vi "Periodic Tasks.vi"(8 "error in":errorcluster) -> ()   [LabVIEW 2020]
doc: "This VI runs in parallel to other tasks. It can contain as many user-defined periodic loops as you need. These can carry out PID or other sorts of timed response."
uses:
  Global Variables/Climber_States.ctl
  <vilib>/Rock Robotics/WPI/Solenoid/WPI_SolenoidValue.ctl
  <vilib>/Rock Robotics/WPI/ThirdParty/REV Robotics/REVLib/Typedef/Spark MAX Control Type.ctl
  <vilib>/Rock Robotics/WPI/ThirdParty/Phoenix-LabVIEW/Motor Controller/Controls/CTRE_Phoenix_MotorControl_ControlMode.ctl
  <vilib>/Rock Robotics/WPI/DriverStation/WPI_DriverStationRobotMode2.ctl
  <vilib>/Rock Robotics/WPI/ThirdParty/Phoenix-LabVIEW/Motor Controller/Controls/CTRE_Phoenix_MotorControl_FeedbackDevice.ctl
  Global Variables/Ball_Routine_States.ctl
  Global Variables/Verification_Delay.ctl
  Global Variables/Shooter_States.ctl
  LabVIEW_is_Under_Control.lib/Util/Toggle/Change Detect.vi
  LabVIEW_is_Under_Control.lib/Util/Toggle/Change Detect Boolean.vi
  <vilib>/Rock Robotics/WPI/Utilities/WPI_GetSetVariantRefNum.vi
  Global Variables/Axes_N_Buttons.vi
  Global Variables/ActuatorsSensors.vi
  Global Variables/StateMachineOperation.vi
  <vilib>/Rock Robotics/Network Tables/NT Write Number.vi
  <vilib>/Rock Robotics/WPI/Solenoid/WPI_SolenoidSetEnum.vi
  Robot Global Data.vi
  <vilib>/Rock Robotics/WPI/ThirdParty/Phoenix-LabVIEW/Motor Controller/Get/CTRE_Phoenix_MotorController_GetSelectedSensorData.vi
  <vilib>/Rock Robotics/Network Tables/NT Write Boolean.vi
  <vilib>/Rock Robotics/Network Tables/NT Write String.vi
panel:
  in  "Robot Control":T1(tab)=enum."Shooter"
  out "Right Current":dbl
  out "Left Current":dbl
  out "Left Current":T2(graph)
  in  "Sensitivity":dbl=1.1
  out "Right Current":T2(graph)
  in  "Reset L":bool
  in  "Reset R":bool
  out "Sensor Position R":dbl=13.714309692382812
  out "Sensor Position L":dbl=5.142850875854492
  out "Shooting?":bool
  out "Applied Output":dbl
  out "ShooterRPM":dbl=352.7285869172389
  out "Voltage":dbl=12.2890625
  out "Output":cluster{"Voltage":dbl}(graph)
  out "Setpoint Shooter":dbl=850.0
  out "PID":cluster{"Setpoint":dbl, "Sensor Position":dbl}(graph)={"Setpoint"=0.0, "Sensor Position"=352.7285869172389}
  in  "PID Constants":T3={"P Gain"=1.5e-05, "I Gain"=0.0, "D Gain"=0.0, "F Gain"=0.00022, "I Zone"=100000.0, "Min Output"=-1.0, "Max Output"=1.0}
  out "RPM Ready?":bool
  in  "SpShooter":dbl=850.0
  in  "Gains":T4={"proportional gain (Kc)"=0.0005, "integral time (Ti, min)"=0.005, "derivative time (Td, min)"=0.0} {"derivative time (Td, min)" format="%.6f"; "integral time (Ti, min)" format="%.6f"; "proportional gain (Kc)" format="%.6f"}
  in  "Range":cluster{"output high":dbl, "output low":dbl}={"output high"=1.0, "output low"=0.0} {"output low" format="%.2f"; "output high" format="%.2f"}
  in  "SpShooter Low Goal":dbl=1000.0
  in  "Hood Low Goal SP":dbl=1000.0
  out "ShooterHoodRPM;":dbl=-0.0
  out "Waveform Chart Hood":cluster{"Shooter Setpoint":dbl, dbl}(graph)={"Shooter Setpoint"=3000.0, -0.0}
  out "Output Chart Hood":cluster{"Percent Output":dbl}(graph)
  in  "I Zone Hood":dbl=1000.0
  in  "kF Hood":dbl=0.005
  in  "D Hood":dbl
  in  "I Hood":dbl
  in  "P Hood":dbl=0.0045
  in  "Neutral to Full Seconds Hood":dbl
  in  "Hood Setpoint Shooter":dbl=3000.0
  out "Setpoint Shooter Hood":dbl=3000.0
  in  "Reset Climber":bool
  out "Climbing State":T5
  out "Climbing?":bool
  out "Sensor Position":dbl
  out "1 Ball only":bool
  out "Discard Left":bool
  out "Discard Right":bool
  out "Overwrite Solenoid":bool
  out "Has 2 Balls":bool
  out "Left Infrared Conveyor":bool
  out "Right Infrared Conveyor":bool
  out "Has Ball Left":bool
  out "Has Ball Right":bool
  out "Opposite Ball Right":bool
  out "Opposite Ball Left":bool
  out "Opposite Color":string="Red"
  out "Ball Color":string="Blue"
  out "RightColor":u32(colorbox)=4488510
  out "LeftColor":u32(colorbox)=4488765
  out "Left Switch Conveyor":bool
  out "Right Switch Conveyor":bool
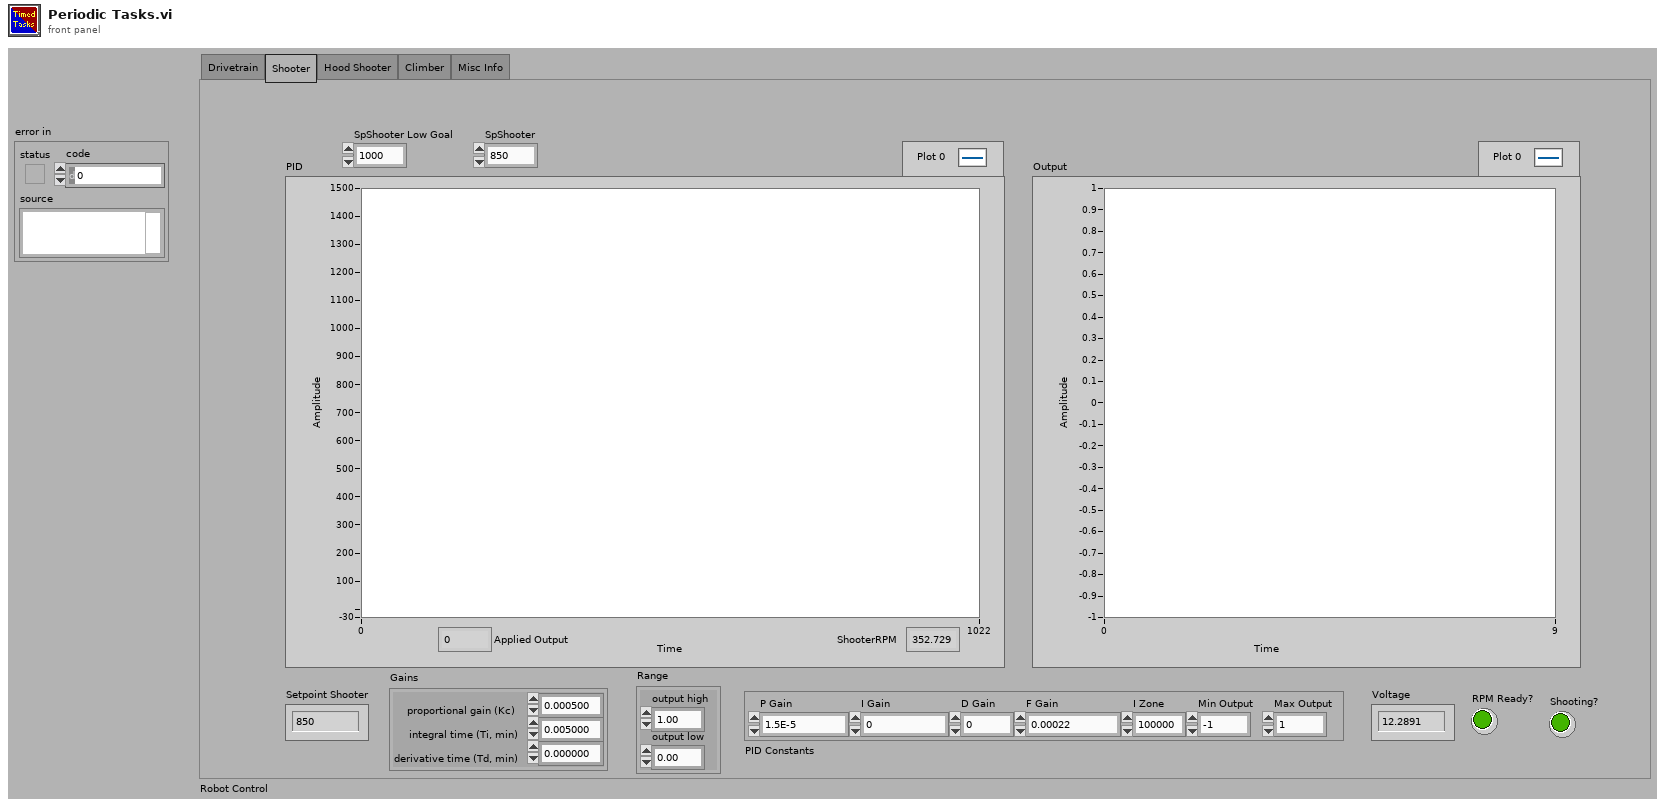
[diagram p1: front panel]
types:
  T1 = enum32{"Drivetrain", "Shooter", "Hood Shooter", "Climber", "Misc Info"}
  T2 = cluster{"current (A)":dbl, "current (A)":dbl, "current (A)":dbl}
  T3 = cluster{"P Gain":dbl, "I Gain":dbl, "D Gain":dbl, "F Gain":dbl, "I Zone":dbl, "Min Output":dbl, "Max Output":dbl}
  T4 = cluster{"proportional gain (Kc)":dbl, "integral time (Ti, min)":dbl, "derivative time (Td, min)":dbl}
  T5 = typedef "Climber_States.ctl" = enum16{"Start Lock", "Release Climber", "Reset Encoder", "Pull Climber", "Lock Pull", "Final Pull", "Lock", "Unspool Release"}
  T6 = typedef "WPI_MotorControlDeviceRef.ctl" = cluster{"DeviceStatus":errorcluster, "Type":T7, "PWM":cluster{"PWM Channel":T8, "DeadBand":T9}, "CAN":cluster{"Device Number":u8, "SetOutput VI Ref":variant, "GetOutput VI Ref":variant, "Enable VI Ref":variant, "Disable VI Ref":variant, "Data":variant}, "Invert":bool, "DIO PWM":cluster{"PWM \"Enable\" Channel":T8, "DIOChannel":T10, "PWM Rate":dbl}}
  T7 = typedef "WPI_MotorControlType.ctl" = enum16{"PWM", "CAN", "DIO PWM"}
  T8 = typedef "FPGA_DIOPWMChannel.ctl" = enum8{"PWM 0", "PWM 1", "PWM 2", "PWM 3", "PWM 4", "PWM 5", "PWM 6", "PWM 7", "PWM 8", "PWM 9", "PWM MXP 0", "PWM MXP 1", "PWM MXP 2", "PWM MXP 3", "PWM MXP 4", "PWM MXP 5", "PWM MXP 6", "PWM MXP 7", "PWM MXP 8", "PWM MXP 9", "Invalid"}
  T9 = typedef "WPI_PWMDeadband.ctl" = cluster{"Name":string, "maxPositivePwm":i32, "minPositivePwm":i32, "centerPwm":i32, "maxNegativePwm":i32, "minNegativePwm":i32, "angularRange":u16}
  T10 = typedef "FPGA_DIOChannel.ctl" = enum8{"DIO 0", "DIO 1", "DIO 2", "DIO 3", "DIO 4", "DIO 5", "DIO 6", "DIO 7", "DIO 8", "DIO 9", "DIO MXP 0", "DIO MXP 1", "DIO MXP 2", "DIO MXP 3", "DIO MXP 4", "DIO MXP 5", "DIO MXP 6", "DIO MXP 7", "DIO MXP 8", "DIO MXP 9", "DIO MXP 10", "DIO MXP 11", "DIO MXP 12", "DIO MXP 13", "DIO MXP 14", "DIO MXP 15", "SPI Port CS1", "SPI Port CS2", "SPI Port CS3", "SPI Port MISO", "SPI Port MOSI", "Invalid"}
  T11 = typedef "WPI_SwitchDevRef.ctl" = cluster{"DevStatus":errorcluster, "DIO Channel":T10, "CntIndex":T12, "Normally Closed":bool}
  T12 = typedef "FPGA_CounterCtrSystemIndex.ctl" = enum8{"Ctr 0", "Ctr 1", "Ctr 2", "Ctr 3", "Ctr 4", "Ctr 5", "Ctr 6", "Ctr 7", "Invalid"}
  T13 = typedef "WPI_DigitalOutputDevRef.ctl" = cluster{"DIO Channel":T10, "DevStatus":errorcluster}
  T14 = typedef "WPI_SolenoidDevRef.ctl" = cluster{"DevStatus":errorcluster, "Pneumatics Control Module":u8, "Forward Solenoid Channel":T15, "Reverse Solenoid Channel":T15}
  T15 = typedef "WPI_SolenoidChannel.ctl" = enum8{"Solenoid 0", "Solenoid 1", "Solenoid 2", "Solenoid 3", "Solenoid 4", "Solenoid 5", "Solenoid 6", "Solenoid 7", "Solenoid 8", "Solenoid 9", "Solenoid 10", "Solenoid 11", "Solenoid 12", "Solenoid 13", "Solenoid 14", "Solenoid 15", "Invalid"}
  T16 = typedef "WPI_CompressorDevRef.ctl" = cluster{"DevStatus":errorcluster, "Pneumatics Control Module":u8}
  T17 = typedef "WPI_SolenoidValue.ctl" = enum16{"Off", "On", "Forward", "Reverse"}
  T18 = typedef "Spark MAX Control Type.ctl" = enum16{"Percent VBus", "Voltage", "Velocity", "Position", "Smart Motion", "Current", "Smart Velocity"}
  T19 = typedef "CTRE_Phoenix_MotorControl_ControlMode.ctl" = u16
  T20 = typedef "WPI_DriverStationRobotMode2.ctl" = enum16{"Autonomous Disabled", "Autonomous Enabled", "Teleop Disabled", "Teleop Enabled", "Disconnected", "Finish", "Test Disabled", "Test Enabled", "Emergency Stopped"}
  T21 = typedef "Color Sensor V3 DevRef.ctl" = cluster{"I2CDevRef":T22}
  T22 = typedef "WPI_I2CDevRef.ctl" = cluster{"DevStatus":errorcluster, "Device Address":u8, "Handle":i32, "I2C Bus":T23}
  T23 = typedef "i2c_bus.ctl" = enum16{"I2C On-Board", "I2C MXP", "Invalid"}
  T24 = typedef "Verification_Delay.ctl" = enum16{"Verifying", "Delayed"}
  T25 = typedef "Ball_Routine_States.ctl" = enum16{"Default", "Dual Intake Collect", "Front Intake Collect", "Rear Intake Collect", "Prepare Shooter", "Shoot", "Climbing", "Opposite Ball Detected", "Low Goal Mode", "Low Goal Shoot"}
  T26 = typedef "WPI_EncoderDevRef.ctl" = cluster{"DevStatus":errorcluster, "EncoderIndex":T27, "CounterIndex":T12, "DistancePerCount":dbl, "Decoding Type":T28}
  T27 = typedef "FPGA_EncoderIdx.ctl" = enum8{"Enc 0", "Enc 1", "Enc 2", "Enc 3", "Enc 4", "Enc 5", "Enc 6", "Enc 7", "Invalid"}
  T28 = typedef "WPI_EncoderType.ctl" = enum16{"1x", "2x", "4x"}
  T29 = typedef "CTRE_Phoenix_MotorControl_FeedbackDevice.ctl" = i8
  T30 = typedef "Shooter_States.ctl" = enum16{"Disabled", "Cruise Velocity", "Shooting Velocity"}
  T31 = cluster{"P Gain":bool, "I Gain":bool, "D Gain":bool, "F Gain":bool, "I Zone":bool, "Min Output":bool, "Max Output":bool}
  T32 = cluster{"Setpoint Shooter":dbl, "Sensor Velocity":dbl}
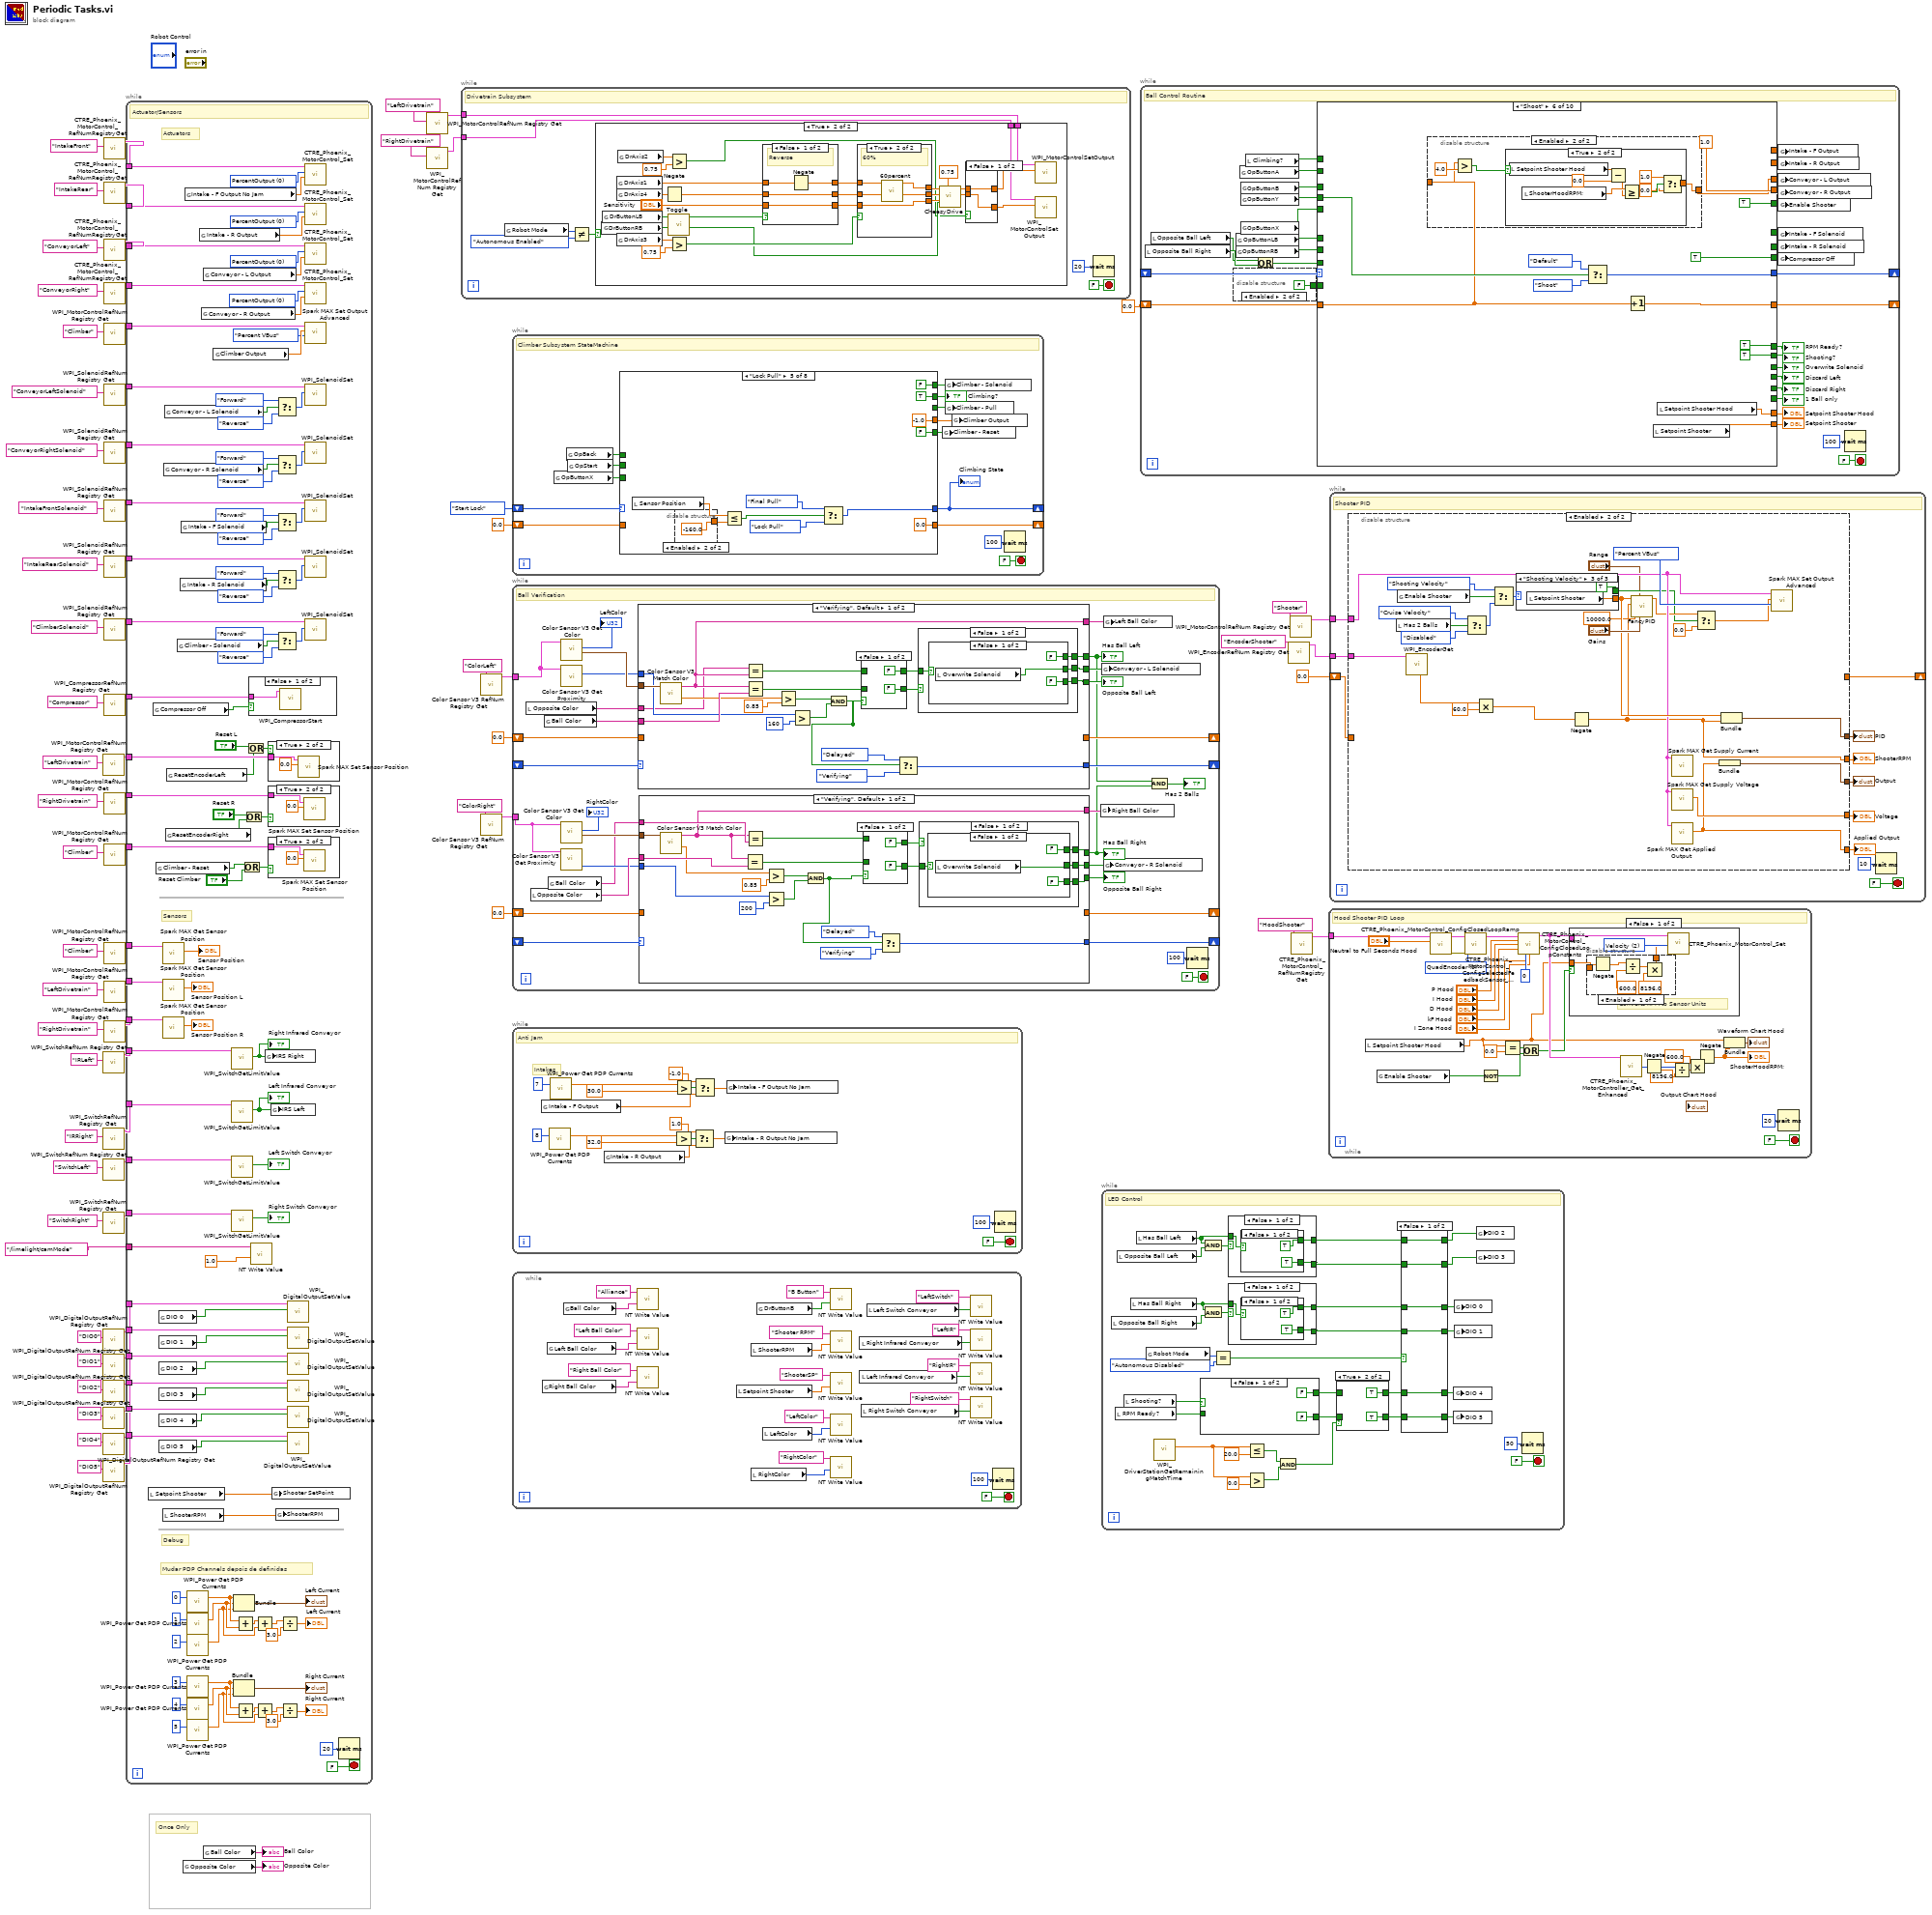
[diagram p0: block diagram]
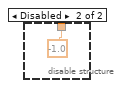
[diagram p2: hidden frame]
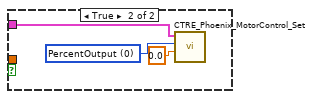
[diagram p3: hidden frame]
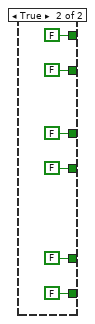
[diagram p4: hidden frame]
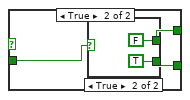
[diagram p6: hidden frame]
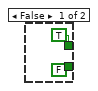
[diagram p7: hidden frame]
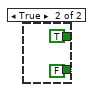
[diagram p8: hidden frame]
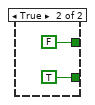
[diagram p9: hidden frame]
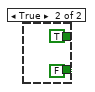
[diagram p10: hidden frame]
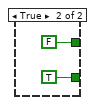
[diagram p11: hidden frame]
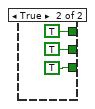
[diagram p13: hidden frame]
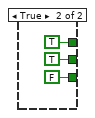
[diagram p14: hidden frame]
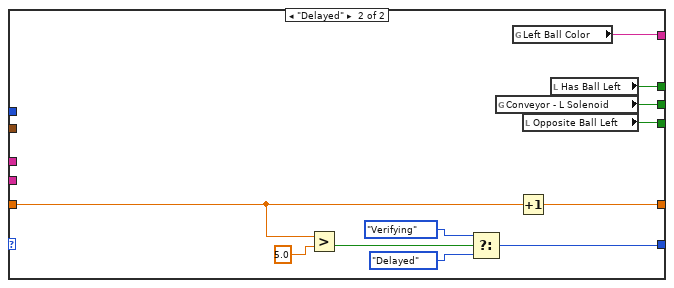
[diagram p15: hidden frame]
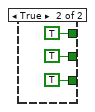
[diagram p17: hidden frame]
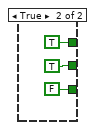
[diagram p18: hidden frame]
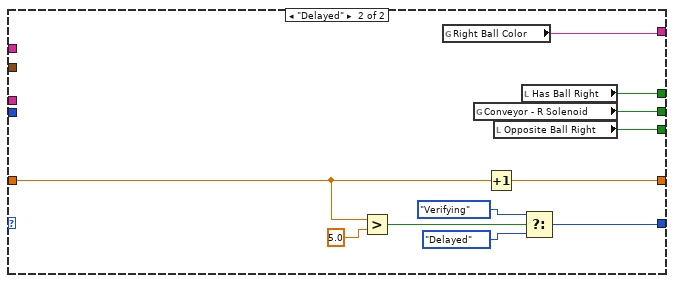
[diagram p19: hidden frame]
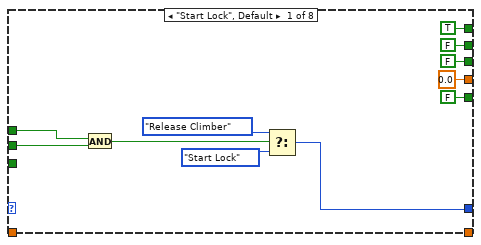
[diagram p20: hidden frame]
diagram:
  # "Once Only"
  n1 = call <vilib>:"WPI_MotorControlRefNum Registry Get.vi"("refnum name"="LeftDrivetrain") -> ("MotorControlDevRef"=w53:T6)  [unwired: 9 in, 1 out]
  n2 = call <vilib>:"WPI_SwitchRefNum Registry Get.vi"("refnum name"="IRLeft") -> ("SwitchDevRef"=w57:T11)  [unwired: 9 in, 1 out]
  n3 = call <vilib>:"WPI_SwitchRefNum Registry Get.vi"("refnum name"="IRRight") -> ("SwitchDevRef"=w56:T11)  [unwired: 9 in, 1 out]
  n4 = call <vilib>:"WPI_SwitchRefNum Registry Get.vi"("refnum name"="SwitchLeft") -> ("SwitchDevRef"=w38:T11)  [unwired: 9 in, 1 out]
  n5 = call <vilib>:"WPI_SwitchRefNum Registry Get.vi"("refnum name"="SwitchRight") -> ("SwitchDevRef"=w37:T11)  [unwired: 9 in, 1 out]
  n6 = call <vilib>:"WPI_DigitalOutputRefNum Registry Get.vi"("refnum name"="DIO0") -> ("DigitalOutputDevRef"=w21:T13)  [unwired: 9 in, 1 out]
  n7 = call <vilib>:"WPI_DigitalOutputRefNum Registry Get.vi"("refnum name"="DIO1") -> ("DigitalOutputDevRef"=w14:T13)  [unwired: 9 in, 1 out]
  n8 = call <vilib>:"WPI_DigitalOutputRefNum Registry Get.vi"("refnum name"="DIO2") -> ("DigitalOutputDevRef"=w13:T13)  [unwired: 9 in, 1 out]
  n9 = call <vilib>:"WPI_DigitalOutputRefNum Registry Get.vi"("refnum name"="DIO3") -> ("DigitalOutputDevRef"=w12:T13)  [unwired: 9 in, 1 out]
  n10 = call <vilib>:"WPI_DigitalOutputRefNum Registry Get.vi"("refnum name"="DIO4") -> ("DigitalOutputDevRef"=w11:T13)  [unwired: 9 in, 1 out]
  n11 = call <vilib>:"WPI_DigitalOutputRefNum Registry Get.vi"("refnum name"="DIO5") -> ("DigitalOutputDevRef"=w10:T13)  [unwired: 9 in, 1 out]
  n12 = call <vilib>:"CTRE_Phoenix_MotorControl_RefNumRegistryGet.vi"("refnum name"="IntakeFront") -> ("PhoenixMotorControlDevRef"=w77:T6)  [unwired: 9 in, 1 out]
  n13 = call <vilib>:"CTRE_Phoenix_MotorControl_RefNumRegistryGet.vi"("refnum name"="IntakeRear") -> ("PhoenixMotorControlDevRef"=w75:T6)  [unwired: 9 in, 1 out]
  n14 = call <vilib>:"CTRE_Phoenix_MotorControl_RefNumRegistryGet.vi"("refnum name"="ConveyorLeft") -> ("PhoenixMotorControlDevRef"=w74:T6)  [unwired: 9 in, 1 out]
  n15 = call <vilib>:"CTRE_Phoenix_MotorControl_RefNumRegistryGet.vi"("refnum name"="ConveyorRight") -> ("PhoenixMotorControlDevRef"=w71:T6)  [unwired: 9 in, 1 out]
  n16 = call <vilib>:"WPI_MotorControlRefNum Registry Get.vi"("refnum name"="Climber") -> ("MotorControlDevRef"=w70:T6)  [unwired: 9 in, 1 out]
  n17 = call <vilib>:"WPI_SolenoidRefNum Registry Get.vi"("refnum name"="ConveyorLeftSolenoid") -> ("SolenoidDevRef"=w69:T14)  [unwired: 9 in, 1 out]
  n18 = call <vilib>:"WPI_SolenoidRefNum Registry Get.vi"("refnum name"="ConveyorRightSolenoid") -> ("SolenoidDevRef"=w68:T14)  [unwired: 9 in, 1 out]
  n19 = call <vilib>:"WPI_SolenoidRefNum Registry Get.vi"("refnum name"="IntakeFrontSolenoid") -> ("SolenoidDevRef"=w67:T14)  [unwired: 9 in, 1 out]
  n20 = call <vilib>:"WPI_SolenoidRefNum Registry Get.vi"("refnum name"="IntakeRearSolenoid") -> ("SolenoidDevRef"=w60:T14)  [unwired: 9 in, 1 out]
  n21 = call <vilib>:"WPI_SolenoidRefNum Registry Get.vi"("refnum name"="ClimberSolenoid") -> ("SolenoidDevRef"=w66:T14)  [unwired: 9 in, 1 out]
  n22 = call <vilib>:"WPI_CompressorRefNum Registry Get.vi"("refnum name"="Compressor") -> ("CompressorDevRef"=w55:T16)  [unwired: 9 in, 1 out]
  n23 = call <vilib>:"WPI_MotorControlRefNum Registry Get.vi"("refnum name"="RightDrivetrain") -> ("MotorControlDevRef"=w54:T6)  [unwired: 9 in, 1 out]
  n24 = call <vilib>:"WPI_MotorControlRefNum Registry Get.vi"("refnum name"="Climber") -> ("MotorControlDevRef"=w48:T6)  [unwired: 9 in, 1 out]
  n25 = call <vilib>:"WPI_MotorControlRefNum Registry Get.vi"("refnum name"="Climber") -> ("MotorControlDevRef"=w46:T6)  [unwired: 9 in, 1 out]
  n26 = call <vilib>:"WPI_MotorControlRefNum Registry Get.vi"("refnum name"="LeftDrivetrain") -> ("MotorControlDevRef"=w40:T6)  [unwired: 9 in, 1 out]
  n27 = call <vilib>:"WPI_MotorControlRefNum Registry Get.vi"("refnum name"="RightDrivetrain") -> ("MotorControlDevRef"=w39:T6)  [unwired: 9 in, 1 out]
  n28 = while {
    tunnel: w77 -> [w183]
    tunnel: w75 -> [w180]
    tunnel: w74 -> [w179]
    tunnel: w71 -> [w178]
    tunnel: w70 -> [w177]
    tunnel: w69 -> [w176]
    tunnel: w68 -> [w175]
    tunnel: w67 -> [w174]
    tunnel: w66 -> [w173]
    tunnel: w60 -> [w168]
    tunnel: w57 -> [w137]
    tunnel: w56 -> [w136]
    tunnel: w55 -> [w134]
    tunnel: w54 -> [w132]
    tunnel: w53 -> [w131]
    tunnel: w48 -> [w130]
    tunnel: w46 -> [w129]
    tunnel: w40 -> [w122]
    tunnel: w39 -> [w121]
    tunnel: w38 -> [w112]
    tunnel: w37 -> [w111]
    tunnel: "/limelight/camMode" ("Name") -> [w99]
    tunnel: w21 -> [w90]
    tunnel: w14 -> [w89]
    tunnel: w13 -> [w88]
    tunnel: w12 -> [w87]
    tunnel: w11 -> [w86]
    tunnel: w10 -> [w85]
    stop <- FALSE stop-if-true
    w93 = T19 0 items=["PercentOutput"=0, "Position"=1, "Velocity"=2, "Current"=3, "Follower"=5, "MotionProfile"=6, "MotionMagic"=7, "MotionProfileArc"=10, "Disabled"=15] ("Control Mode")
    w94 = T19 0 items=["PercentOutput"=0, "Position"=1, "Velocity"=2, "Current"=3, "Follower"=5, "MotionProfile"=6, "MotionMagic"=7, "MotionProfileArc"=10, "Disabled"=15] ("Control Mode")
    w102 = T19 0 items=["PercentOutput"=0, "Position"=1, "Velocity"=2, "Current"=3, "Follower"=5, "MotionProfile"=6, "MotionMagic"=7, "MotionProfileArc"=10, "Disabled"=15] ("Control Mode")
    w181 = T19 0 items=["PercentOutput"=0, "Position"=1, "Velocity"=2, "Current"=3, "Follower"=5, "MotionProfile"=6, "MotionMagic"=7, "MotionProfileArc"=10, "Disabled"=15] ("Control Mode")
    # "Debug"
    # "Mudar PDP Channels depois de definidas"
    # "Sensors"
    # "Actuators"
    # "Actuator/Sensors"
    n29 = local read "Setpoint Shooter"() -> (w78:dbl)
    n30 = global read "ActuatorsSensors.vi" "Compressor Off"() -> (w133:bool)
    n31 = global read "StateMachineOperation.vi" "Climber - Reset"() -> (w124:bool)
    n32 = global read "ActuatorsSensors.vi" "DIO 0"() -> (w84:bool)
    n33 = global read "ActuatorsSensors.vi" "DIO 1"() -> (w83:bool)
    n34 = global read "ActuatorsSensors.vi" "DIO 2"() -> (w82:bool)
    n35 = global read "ActuatorsSensors.vi" "DIO 3"() -> (w81:bool)
    n36 = global read "ActuatorsSensors.vi" "DIO 4"() -> (w80:bool)
    n37 = global read "ActuatorsSensors.vi" "DIO 5"() -> (w79:bool)
    n38 = call <vilib>:"Spark MAX Get Sensor Position.vi"("MotorControlDevRef in"=w129) -> ("Sensor Position"=→"Sensor Position":dbl)  [unwired: 7 in, 3 out]
    n39 = call <vilib>:"Spark MAX Get Sensor Position.vi"("MotorControlDevRef in"=w122) -> ("Sensor Position"=→"Sensor Position L":dbl)  [unwired: 7 in, 3 out]
    n40 = call <vilib>:"Spark MAX Get Sensor Position.vi"("MotorControlDevRef in"=w121) -> ("Sensor Position"=→"Sensor Position R":dbl)  [unwired: 7 in, 3 out]
    n41 = local read "ShooterRPM"() -> (w135:dbl)
    n42 = global read "ActuatorsSensors.vi" "Conveyor - R Solenoid"() -> (w139:bool)
    n43 = global read "ActuatorsSensors.vi" "Conveyor - L Solenoid"() -> (w138:bool)
    n44 = global read "ActuatorsSensors.vi" "ResetEncoderRight"() -> (w118:bool)
    n45 = global read "ActuatorsSensors.vi" "ResetEncoderLeft"() -> (w114:bool)
    n46 = global read "ActuatorsSensors.vi" "Climber - Solenoid"() -> (w107:bool)
    n47 = global read "ActuatorsSensors.vi" "Intake - R Solenoid"() -> (w104:bool)
    n48 = global read "ActuatorsSensors.vi" "Intake - F Solenoid"() -> (w169:bool)
    n49 = global read "ActuatorsSensors.vi" "Intake - F Output No Jam"() -> (w182:dbl)
    n50 = call <vilib>:"WPI_Power Get PDP Currents.vi"("PDP Channel"=0) -> ("current (A)"=w163:dbl)  [unwired: 12 in, 2 out]
    n51 = call <vilib>:"WPI_Power Get PDP Currents.vi"("PDP Channel"=1) -> ("current (A)"=w162:dbl)  [unwired: 12 in, 2 out]
    n52 = call <vilib>:"WPI_Power Get PDP Currents.vi"("PDP Channel"=2) -> ("current (A)"=w160:dbl)  [unwired: 12 in, 2 out]
    n53 = call <vilib>:"WPI_Power Get PDP Currents.vi"("PDP Channel"=3) -> ("current (A)"=w155:dbl)  [unwired: 12 in, 2 out]
    n54 = call <vilib>:"WPI_Power Get PDP Currents.vi"("PDP Channel"=4) -> ("current (A)"=w154:dbl)  [unwired: 12 in, 2 out]
    n55 = call <vilib>:"WPI_Power Get PDP Currents.vi"("PDP Channel"=5) -> ("current (A)"=w152:dbl)  [unwired: 12 in, 2 out]
    n56 = global read "ActuatorsSensors.vi" "Intake - R Output"() -> (w101:dbl)
    n57 = global read "ActuatorsSensors.vi" "Conveyor - R Output"() -> (w91:dbl)
    n58 = global read "ActuatorsSensors.vi" "Conveyor - L Output"() -> (w92:dbl)
    n59 = global read "ActuatorsSensors.vi" "Climber Output"() -> (w127:dbl)
    n60 = call <vilib>:"WPI_SwitchGetLimitValue.vi"("SwitchDevRef"=w137) -> ("Switch Pressed"=w98:bool)  [unwired: 8 in, 2 out]
    "Right Infrared Conveyor" <- w98
    n61 = call <vilib>:"WPI_SwitchGetLimitValue.vi"("SwitchDevRef"=w136) -> ("Switch Pressed"=w97:bool)  [unwired: 8 in, 2 out]
    "Left Infrared Conveyor" <- w97
    n62 = call <vilib>:"WPI_SwitchGetLimitValue.vi"("SwitchDevRef"=w112) -> ("Switch Pressed"=→"Left Switch Conveyor":bool)  [unwired: 8 in, 2 out]
    n63 = call <vilib>:"WPI_SwitchGetLimitValue.vi"("SwitchDevRef"=w111) -> ("Switch Pressed"=→"Right Switch Conveyor":bool)  [unwired: 8 in, 2 out]
    n64 = Bundle("current (A)"=w163, "current (A)"=w162, "current (A)"=w160) -> (→"Left Current":T2)  [unwired: 1 in]
    n65 = Bundle("current (A)"=w155, "current (A)"=w154, "current (A)"=w152) -> (→"Right Current":T2)  [unwired: 1 in]
    n66 = Add(x=w163, y=w162) -> (x+y=w161:dbl)
    n67 = Add(x=w155, y=w154) -> (x+y=w153:dbl)
    n68 = Or(x=w124, y="Reset Climber") -> (x .or. y?=w126:bool)
    n69 = Or(x="Reset R", y=w118) -> (x .or. y?=w117:bool)
    n70 = Or(x="Reset L", y=w114) -> (x .or. y?=w115:bool)
    n71 = case shown="False" w133 {
      tunnel: w134 -> [w192 w193]
      frame False {
        n72 = call <vilib>:"WPI_CompressorStart.vi"("CompressorDevRef"=w192) -> ()  [unwired: 9 in, 2 out]
      }
      frame True {
        n73 = call <vilib>:"WPI_CompressorStop.vi"("CompressorDevRef"=w193) -> ()  [unwired: 9 in, 2 out]
      }
    }
    n74 = call-poly <vilib>:"NT Write Value.vi"("Numeric"=1.0, "Name"=w99) -> ()  [unwired: 9 in, 1 out]
    n75 = Add(x=w161, y=w160) -> (x+y=w159:dbl)
    n76 = Add(x=w153, y=w152) -> (x+y=w151:dbl)
    n77 = global write "ActuatorsSensors.vi" "IRS Right"(w98) -> ()
    n78 = case shown="True" w115 {
      tunnel: w131 -> [_ w188]
      frame False {
      }
      frame True {
        n79 = call <vilib>:"Spark MAX Set Sensor Position.vi"("Position"=0.0, "MotorControlDeviceRef"=w188) -> ()  [unwired: 8 in, 2 out]
      }
    }
    n80 = case shown="True" w117 {
      tunnel: w132 -> [_ w190]
      frame False {
      }
      frame True {
        n81 = call <vilib>:"Spark MAX Set Sensor Position.vi"("Position"=0.0, "MotorControlDeviceRef"=w190) -> ()  [unwired: 8 in, 2 out]
      }
    }
    n82 = case shown="True" w126 {
      tunnel: w130 -> [_ w186]
      frame False {
      }
      frame True {
        n83 = call <vilib>:"Spark MAX Set Sensor Position.vi"("Position"=0.0, "MotorControlDeviceRef"=w186) -> ()  [unwired: 8 in, 2 out]
      }
    }
    n84 = global write "ActuatorsSensors.vi" "IRS Left"(w97) -> ()
    n85 = global write "ActuatorsSensors.vi" "Shooter SetPoint"(w78) -> ()
    n86 = global write "ActuatorsSensors.vi" "ShooterRPM"(w135) -> ()
    n87 = Select(t=WPI_SolenoidValue."Forward" ("Value"), s=w138, f=WPI_SolenoidValue."Reverse" ("Value")) -> (s? t:f=w141:T17)
    n88 = Select(t=WPI_SolenoidValue."Forward" ("Value"), s=w139, f=WPI_SolenoidValue."Reverse" ("Value")) -> (s? t:f=w140:T17)
    n89 = Select(t=WPI_SolenoidValue."Forward" ("Value"), s=w169, f=WPI_SolenoidValue."Reverse" ("Value")) -> (s? t:f=w170:T17)
    n90 = Select(t=WPI_SolenoidValue."Forward" ("Value"), s=w104, f=WPI_SolenoidValue."Reverse" ("Value")) -> (s? t:f=w103:T17)
    n91 = Select(t=WPI_SolenoidValue."Forward" ("Value"), s=w107, f=WPI_SolenoidValue."Reverse" ("Value")) -> (s? t:f=w108:T17)
    n92 = Divide(x=w159, y=3.0) -> (x/y=→"Left Current":dbl)
    n93 = Divide(x=w151, y=3.0) -> (x/y=→"Right Current":dbl)
    n94 = call <vilib>:"WPI_DigitalOutputSetValue.vi"("Value"=w84, "DigitalOutputDevRef"=w90) -> ()  [unwired: 8 in, 2 out]
    n95 = call <vilib>:"WPI_DigitalOutputSetValue.vi"("Value"=w83, "DigitalOutputDevRef"=w89) -> ()  [unwired: 8 in, 2 out]
    n96 = call <vilib>:"WPI_DigitalOutputSetValue.vi"("Value"=w82, "DigitalOutputDevRef"=w88) -> ()  [unwired: 8 in, 2 out]
    n97 = call <vilib>:"WPI_DigitalOutputSetValue.vi"("Value"=w81, "DigitalOutputDevRef"=w87) -> ()  [unwired: 8 in, 2 out]
    n98 = call <vilib>:"WPI_DigitalOutputSetValue.vi"("Value"=w80, "DigitalOutputDevRef"=w86) -> ()  [unwired: 8 in, 2 out]
    n99 = call <vilib>:"WPI_DigitalOutputSetValue.vi"("Value"=w79, "DigitalOutputDevRef"=w85) -> ()  [unwired: 8 in, 2 out]
    n100 = call <vilib>:"CTRE_Phoenix_MotorControl_Set.vi"("Output"=w182, "Control Mode"=w181, "PhoenixMotorControlDevRef"=w183) -> ()  [unwired: 7 in, 2 out]
    n101 = call <vilib>:"CTRE_Phoenix_MotorControl_Set.vi"("Output"=w101, "Control Mode"=w102, "PhoenixMotorControlDevRef"=w180) -> ()  [unwired: 7 in, 2 out]
    n102 = call <vilib>:"CTRE_Phoenix_MotorControl_Set.vi"("Output"=w92, "Control Mode"=w93, "PhoenixMotorControlDevRef"=w179) -> ()  [unwired: 7 in, 2 out]
    n103 = call <vilib>:"CTRE_Phoenix_MotorControl_Set.vi"("Output"=w91, "Control Mode"=w94, "PhoenixMotorControlDevRef"=w178) -> ()  [unwired: 7 in, 2 out]
    n104 = call <vilib>:"Spark MAX Set Output Advanced.vi"("Control Mode"=Spark_MAX_Control_Type."Percent VBus", "Setpoint"=w127, "MotorControlDevRef"=w177) -> ()  [unwired: 7 in, 2 out]
    n105 = call-poly <vilib>:"WPI_SolenoidSet.vi"("Value"=w141, "SolenoidDevRef"=w176) -> ()  [unwired: 8 in, 2 out]
    n106 = call-poly <vilib>:"WPI_SolenoidSet.vi"("Value"=w140, "SolenoidDevRef"=w175) -> ()  [unwired: 8 in, 2 out]
    n107 = call-poly <vilib>:"WPI_SolenoidSet.vi"("Value"=w170, "SolenoidDevRef"=w174) -> ()  [unwired: 8 in, 2 out]
    n108 = call-poly <vilib>:"WPI_SolenoidSet.vi"("Value"=w103, "SolenoidDevRef"=w168) -> ()  [unwired: 8 in, 2 out]
    n109 = call-poly <vilib>:"WPI_SolenoidSet.vi"("Value"=w108, "SolenoidDevRef"=w173) -> ()  [unwired: 8 in, 2 out]
    n110 = Wait (ms)(milliseconds to wait=u32 20) -> ()  [unwired: 1 out]
  }
  n111 = global read "StateMachineOperation.vi" "Opposite Color"() -> (→"Opposite Color":string)
  n112 = global read "StateMachineOperation.vi" "Ball Color"() -> (→"Ball Color":string)
  n113 = call <vilib>:"WPI_MotorControlRefNum Registry Get.vi"("refnum name"="LeftDrivetrain") -> ("MotorControlDevRef"=w6:T6)  [unwired: 9 in, 1 out]
  n114 = call <vilib>:"WPI_MotorControlRefNum Registry Get.vi"("refnum name"="RightDrivetrain") -> ("MotorControlDevRef"=w5:T6)  [unwired: 9 in, 1 out]
  n115 = while {
    tunnel: w6 -> [w195]
    tunnel: w5 -> [w194]
    stop <- FALSE stop-if-true
    # "Drivetrain Subsystem"
    n116 = global read "Robot Global Data.vi" "Robot Mode"() -> (w198:T20)
    n117 = Not Equal?(x=w198, y=WPI_DriverStationRobotMode2."Autonomous Enabled" ("Robot Mode")) -> (x != y?=w196:bool)
    n118 = case shown="True" w196 {
      tunnel: w195 -> [_ w211]
      tunnel: w194 -> [_ w202]
      frame False {
      }
      frame True {
        n119 = global read "Axes_N_Buttons.vi" "DrButtonRB"() -> (w212:bool)
        n120 = global read "Axes_N_Buttons.vi" "DrButtonLB"() -> (w224:bool)
        n121 = global read "Axes_N_Buttons.vi" "DrAxis1"() -> (w207:dbl)
        n122 = global read "Axes_N_Buttons.vi" "DrAxis4"() -> (w225:dbl)
        n123 = global read "Axes_N_Buttons.vi" "DrAxis3"() -> (w215:dbl)
        n124 = global read "Axes_N_Buttons.vi" "DrAxis2"() -> (w210:dbl)
        n125 = Negate(x=w225) -> (-x=w208:dbl)
        n126 = call "Toggle.vi"("In"=w224) -> ("Toggled"=w223:bool)  [unwired: 10 in]
        n127 = Greater?(x=w215, y=0.75) -> (0:w213:bool)
        n128 = Greater?(x=w210, y=0.75) -> (0:w206:bool)
        n129 = case shown="False" w223 {
          tunnel: w207 -> [w240 w242]
          tunnel: w208 -> [w239 w243]
          tunnel: "Sensitivity" -> [w241 w244]
          tunnel: [w241 w244] -> w221
          tunnel: [w238 w242] -> w219
          tunnel: [w239 w243] -> w220
          frame False {
            # "Reverse"
            n130 = Negate(x=w240) -> (-x=w238:dbl)
          }
          frame True {
            # "Reverse"
          }
        }
        n131 = case shown="True" w213 {
          tunnel: w221 -> [w231 w237]
          tunnel: w220 -> [w232 w236]
          tunnel: w219 -> [w233 w235]
          tunnel: [w231 w237] -> w218
          tunnel: [w232 w236] -> w217
          tunnel: [w233 w234] -> w216
          frame False {
            # "60%"
          }
          frame True {
            # "60%"
            n132 = call "60percent.vi"("In"=w235) -> ("Out"=w234:dbl)  [unwired: 10 in]
          }
        }
        n133 = call "CheesyDrive.vi"("Quickturn"=w212, "WheelNonLinearity"=0.75, "Sensitivty"=w218, "Wheel"=w217, "Throttle"=w216) -> ("Right PWM"=w204:dbl, "Left PWM"=w205:dbl)  [unwired: 5 in]
        n134 = case shown="False" w206 {
          tunnel: w205 -> [w228 _]
          tunnel: w204 -> [w227 _]
          tunnel: [w228 0.06 ("Left PWM")] -> w203
          tunnel: [w227 0.06 ("Right PWM")] -> w201
          frame False {
          }
          frame True {
          }
        }
        n135 = call <vilib>:"WPI_MotorControlSetOutput.vi"("Output"=w203, "MotorControlDevRef"=w211) -> ()  [unwired: 7 in, 3 out]
        n136 = call <vilib>:"WPI_MotorControlSetOutput.vi"("Output"=w201, "MotorControlDevRef"=w202) -> ()  [unwired: 7 in, 3 out]
      }
    }
    n137 = Wait (ms)(milliseconds to wait=u32 20) -> ()  [unwired: 1 out]
  }
  n138 = call <vilib>:"Color Sensor V3 RefNum Registry Get.vi"("refnum name"="ColorLeft") -> ("ColorSensorDevRef"=w30:T21)  [unwired: 9 in, 1 out]
  n139 = call <vilib>:"Color Sensor V3 RefNum Registry Get.vi"("refnum name"="ColorRight") -> ("ColorSensorDevRef"=w29:T21)  [unwired: 9 in, 1 out]
  n140 = while {
    shift-right: [w253] -> _
    shift-left: Climber_States."Start Lock" ("Enum") -> [w255]
    shift-right: [w245] -> _
    shift-left: 0.0 ("y") -> [w246]
    stop <- FALSE stop-if-true
    # "Climber Subsystem StateMachine"
    n141 = global read "Axes_N_Buttons.vi" "OpButtonX"() -> (w251:bool)
    n142 = global read "Axes_N_Buttons.vi" "OpBack"() -> (w256:bool)
    n143 = global read "Axes_N_Buttons.vi" "OpStart"() -> (w249:bool)
    n144 = case shown="\"Lock Pull\"" w255 {
      tunnel: w256 -> [w269 _ _ _ _ _ w327 _]
      tunnel: [TRUE ("ClimberSolenoid") FALSE ("ClimberSolenoid") _ FALSE ("ClimberSolenoid") FALSE ("ClimberSolenoid") TRUE ("ClimberSolenoid") TRUE ("ClimberSolenoid") FALSE ("ClimberSolenoid")] -> w252
      tunnel: [FALSE ("Climbing?") TRUE ("Climbing?") TRUE ("Climbing?") TRUE ("Climbing?") TRUE ("Climbing?") TRUE ("Climbing?") FALSE ("Climbing?") TRUE ("Climbing?")] -> w254
      tunnel: [w265 w273 w281 w292 w307 w320 w325 w337] -> w253
      tunnel: w251 -> [_ w272 _ _ _ _ _ w338]
      tunnel: [FALSE FALSE _ TRUE _ _ _ _] -> w250
      tunnel: w249 -> [w261 _ _ _ _ _ w326 _]
      tunnel: [0.0 ("y") _ _ -1.0 ("OpAxis1") -1.0 ("OpAxis1") -1.0 ("OpAxis1") 0.0 ("OpAxis1") w344] -> w248
      tunnel: [FALSE ("Climber - Pull") FALSE ("Climber - Pull") TRUE ("Climber - Pull") FALSE ("Climber - Pull") FALSE ("Climber - Pull") FALSE ("Climber - Pull") FALSE ("Climber - Pull") FALSE ("Climber - Pull")] -> w247
      tunnel: [_ _ w285 _ 0.0 w322 _ _] -> w245
      tunnel: w246 -> [_ _ w284 _ _ w321 _ _]
      frame "Start Lock", Default {
        n145 = And(x=w269, y=w261) -> (x .and. y?=w268:bool)
        n146 = Select(t=Climber_States."Release Climber" ("Enum"), s=w268, f=Climber_States."Start Lock" ("Enum")) -> (s? t:f=w265:T5)
      }
      frame "Release Climber" {
        n147 = Select(t=Climber_States."Reset Encoder" ("Enum"), s=w272, f=Climber_States."Release Climber" ("Enum")) -> (s? t:f=w273:T5)
      }
      frame "Reset Encoder" {
        n148 = Greater?(x=w284, y=1.0) -> (0:w282:bool)
        n149 = Increment(x=w284) -> (x+1=w285:dbl)
        n150 = Select(t=Climber_States."Pull Climber" ("Enum"), s=w282, f=Climber_States."Reset Encoder" ("Enum")) -> (s? t:f=w281:T5)
      }
      frame "Pull Climber" {
        n151 = local read "Sensor Position"() -> (w291:dbl)
        n152 = disable-structure shown="Enabled" {
          disable-tunnel: [-99.0 ("y") -115.0 ("y")] -> w288
          frame Disabled {
          }
          frame Enabled {
          }
        }
        n153 = Less Or Equal?(x=w291, y=w288) -> (x <= y?=w290:bool)
        n154 = Select(t=Climber_States."Lock Pull" ("Enum"), s=w290, f=Climber_States."Pull Climber" ("Enum")) -> (s? t:f=w292:T5)
      }
      frame "Lock Pull" {
        n155 = local read "Sensor Position"() -> (w309:dbl)
        n156 = disable-structure shown="Enabled" {
          disable-tunnel: [-122.5 ("y") -160.0 ("y")] -> w308
          frame Disabled {
          }
          frame Enabled {
          }
        }
        n157 = Less Or Equal?(x=w309, y=w308) -> (x <= y?=w304:bool)
        n158 = Select(t=Climber_States."Final Pull" ("Enum"), s=w304, f=Climber_States."Lock Pull" ("Enum")) -> (s? t:f=w307:T5)
      }
      frame "Final Pull" {
        n159 = Greater?(x=w321, y=1.0) -> (0:w319:bool)
        n160 = Select(t=Climber_States."Lock" ("Enum"), s=w319, f=Climber_States."Final Pull" ("Enum")) -> (s? t:f=w320:T5)
        n161 = Increment(x=w321) -> (x+1=w322:dbl)
      }
      frame "Lock" {
        n162 = And(x=w327, y=w326) -> (x .and. y?=w330:bool)
        n163 = Select(t=Climber_States."Unspool Release" ("Enum"), s=w330, f=Climber_States."Lock" ("Enum")) -> (s? t:f=w325:T5)
      }
      frame "Unspool Release" {
        n164 = local read "Sensor Position"() -> (w347:dbl)
        n165 = local read "Sensor Position"() -> (w349:dbl)
        n166 = Greater Or Equal?(x=w349, y=-1.0) -> (x >= y?=w336:bool)
        n167 = Greater Or Equal?(x=w347, y=-10.0) -> (x >= y?=w335:bool)
        n168 = Select(t=0.2, s=w335, f=1.0) -> (s? t:f=w343:dbl)
        n169 = Select(t=Climber_States."Reset Encoder" ("Enum"), s=w338, f=Climber_States."Unspool Release" ("Enum")) -> (s? t:f=w337:T5)
        n170 = Select(t=0.0, s=w336, f=w343) -> (s? t:f=w344:dbl)
      }
    }
    "Climbing?" <- w254
    "Climbing State" <- w253
    n171 = global write "StateMachineOperation.vi" "Climber - Reset"(w247) -> ()
    n172 = global write "ActuatorsSensors.vi" "Climber - Solenoid"(w252) -> ()
    n173 = global write "StateMachineOperation.vi" "Climber - Pull"(w250) -> ()
    n174 = global write "ActuatorsSensors.vi" "Climber Output"(w248) -> ()
    n175 = Wait (ms)(milliseconds to wait=u32 100) -> ()  [unwired: 1 out]
  }
  n176 = while {
    tunnel: w30 -> [w373]
    tunnel: w29 -> [w372]
    shift-right: [w374] -> _
    shift-left: _ -> [w364]
    shift-right: [w362] -> _
    shift-left: 0.0 ("y") -> [w363]
    shift-right: [w357] -> _
    shift-left: _ -> [w358]
    shift-right: [w355] -> _
    shift-left: 0.0 ("y") -> [w356]
    stop <- FALSE stop-if-true
    # "Ball Verification"
    n177 = local read "Opposite Color"() -> (w361:string)
    n178 = local read "Opposite Color"() -> (w377:string)
    n179 = global read "StateMachineOperation.vi" "Ball Color"() -> (w378:string)
    n180 = global read "StateMachineOperation.vi" "Ball Color"() -> (w360:string)
    n181 = call <vilib>:"Color Sensor V3 Get Color.vi"("ColorSensorDevRef"=w372) -> ("Normalized Color"=w375:cluster{"R":dbl, "G":dbl, "B":dbl}, "Color"=→"RightColor":u32)  [unwired: 7 in, 2 out]
    n182 = call <vilib>:"Color Sensor V3 Get Proximity.vi"("ColorSensorDevRef"=w372) -> ("Proximity"=w371:u16)  [unwired: 8 in, 2 out]
    n183 = call <vilib>:"Color Sensor V3 Get Color.vi"("ColorSensorDevRef"=w373) -> ("Normalized Color"=w376:cluster{"R":dbl, "G":dbl, "B":dbl}, "Color"=→"LeftColor":u32)  [unwired: 7 in, 2 out]
    n184 = call <vilib>:"Color Sensor V3 Get Proximity.vi"("ColorSensorDevRef"=w373) -> ("Proximity"=w370:u16)  [unwired: 8 in, 2 out]
    n185 = case shown="\"Verifying\", Default" w358 {
      tunnel: w378 -> [w403 _]
      tunnel: w376 -> [w402 _]
      tunnel: w370 -> [w401 _]
      tunnel: [w400 w423] -> w368
      tunnel: [w399 w424] -> w367
      tunnel: [w398 w422] -> w352
      tunnel: [w392 w425] -> w365
      tunnel: w361 -> [w388 _]
      tunnel: [w383 w426] -> w357
      tunnel: [_ w431] -> w355
      tunnel: w356 -> [_ w427]
      frame "Verifying", Default {
        n186 = call <vilib>:"Color Sensor V3 Match Color.vi"("Measured Color"=w402) -> ("Confidence"=w397:dbl, "Matched Color Name"=w392:string)  [unwired: 8 in, 1 out]
        n187 = Equal?(x=w388, y=w392) -> (x = y?=w393:bool)
        n188 = Equal?(x=w392, y=w403) -> (x = y?=w395:bool)
        n189 = Greater?(x=w397, y=0.85) -> (0:w389:bool)
        n190 = Greater?(x=w401, y=u16 160) -> (0:w387:bool)
        n191 = And(x=w389, y=w387) -> (x .and. y?=w384:bool)
        n192 = case shown="False" w384 {
          tunnel: [FALSE w407] -> w394
          tunnel: w393 -> [_ w407]
          tunnel: w395 -> [_ w406]
          tunnel: [FALSE w406] -> w396
          frame False {
          }
          frame True {
          }
        }
        n193 = Select(t=Verification_Delay."Delayed" ("Verification Delay State"), s=w384, f=Verification_Delay."Verifying" ("Verification Delay State")) -> (s? t:f=w383:T24)
        n194 = case shown="False" w396 {
          tunnel: w394 -> [w411 _]
          tunnel: [w409 FALSE ("Opposite Ball?")] -> w400
          tunnel: [w410 TRUE ("Conveyor - L Solenoid")] -> w399
          tunnel: [w408 TRUE ("Has Ball Left")] -> w398
          frame False {
            n195 = case shown="False" w411 {
              tunnel: [w412 TRUE ("Conveyor - L Solenoid")] -> w410
              tunnel: [FALSE ("Opposite Ball?") TRUE ("Opposite Ball?")] -> w409
              tunnel: [FALSE ("Has Ball Left") TRUE ("Has Ball Left")] -> w408
              frame False {
                n196 = local read "Overwrite Solenoid"() -> (w412:bool)
              }
              frame True {
              }
            }
          }
          frame True {
          }
        }
      }
      frame "Delayed" {
        n197 = Greater?(x=w427, y=5.0) -> (0:w429:bool)
        n198 = Select(t=Verification_Delay."Verifying" ("Verification Delay State"), s=w429, f=Verification_Delay."Delayed" ("Verification Delay State")) -> (s? t:f=w426:T24)
        n199 = global read "ActuatorsSensors.vi" "Conveyor - L Solenoid"() -> (w424:bool)
        n200 = global read "StateMachineOperation.vi" "Left Ball Color"() -> (w425:string)
        n201 = Increment(x=w427) -> (x+1=w431:dbl)
        n202 = local read "Opposite Ball Left"() -> (w423:bool)
        n203 = local read "Has Ball Left"() -> (w422:bool)
      }
    }
    "Opposite Ball Left" <- w368
    "Has Ball Left" <- w352
    n204 = case shown="\"Verifying\", Default" w364 {
      tunnel: w377 -> [w452 _]
      tunnel: w375 -> [w451 _]
      tunnel: [w450 w474] -> w374
      tunnel: w371 -> [w449 _]
      tunnel: [w448 w472] -> w369
      tunnel: [w447 w470] -> w366
      tunnel: [w446 w471] -> w353
      tunnel: [_ w480] -> w362
      tunnel: w363 -> [_ w479]
      tunnel: w360 -> [w434 _]
      tunnel: [w432 w473] -> w359
      frame "Verifying", Default {
        n205 = call <vilib>:"Color Sensor V3 Match Color.vi"("Measured Color"=w451) -> ("Confidence"=w441:dbl, "Matched Color Name"=w432:string)  [unwired: 8 in, 1 out]
        n206 = Equal?(x=w432, y=w452) -> (x = y?=w444:bool)
        n207 = Equal?(x=w432, y=w434) -> (x = y?=w442:bool)
        n208 = Greater?(x=w441, y=0.85) -> (0:w437:bool)
        n209 = Greater?(x=w449, y=u16 200) -> (0:w435:bool)
        n210 = And(x=w437, y=w435) -> (x .and. y?=w433:bool)
        n211 = case shown="False" w433 {
          tunnel: [FALSE w456] -> w443
          tunnel: w442 -> [_ w456]
          tunnel: [FALSE w455] -> w445
          tunnel: w444 -> [_ w455]
          frame False {
          }
          frame True {
          }
        }
        n212 = Select(t=Verification_Delay."Delayed" ("Verification Delay State"), s=w433, f=Verification_Delay."Verifying" ("Verification Delay State")) -> (s? t:f=w450:T24)
        n213 = case shown="False" w443 {
          tunnel: w445 -> [w460 _]
          tunnel: [w459 TRUE ("Conveyor - L Solenoid")] -> w448
          tunnel: [w458 FALSE ("Opposite Ball?")] -> w447
          tunnel: [w457 TRUE ("Has Ball Right")] -> w446
          frame False {
            n214 = case shown="False" w460 {
              tunnel: [w461 TRUE ("Conveyor - L Solenoid")] -> w459
              tunnel: [FALSE ("Opposite Ball?") TRUE ("Opposite Ball?")] -> w458
              tunnel: [FALSE ("Has Ball Right") TRUE ("Has Ball Right")] -> w457
              frame False {
                n215 = local read "Overwrite Solenoid"() -> (w461:bool)
              }
              frame True {
              }
            }
          }
          frame True {
          }
        }
      }
      frame "Delayed" {
        n216 = Greater?(x=w479, y=5.0) -> (0:w477:bool)
        n217 = global read "StateMachineOperation.vi" "Right Ball Color"() -> (w473:string)
        n218 = global read "ActuatorsSensors.vi" "Conveyor - R Solenoid"() -> (w472:bool)
        n219 = Increment(x=w479) -> (x+1=w480:dbl)
        n220 = local read "Opposite Ball Right"() -> (w470:bool)
        n221 = local read "Has Ball Right"() -> (w471:bool)
        n222 = Select(t=Verification_Delay."Verifying" ("Verification Delay State"), s=w477, f=Verification_Delay."Delayed" ("Verification Delay State")) -> (s? t:f=w474:T24)
      }
    }
    "Opposite Ball Right" <- w366
    "Has Ball Right" <- w353
    n223 = global write "StateMachineOperation.vi" "Right Ball Color"(w359) -> ()
    n224 = global write "ActuatorsSensors.vi" "Conveyor - L Solenoid"(w367) -> ()
    n225 = global write "ActuatorsSensors.vi" "Conveyor - R Solenoid"(w369) -> ()
    n226 = global write "StateMachineOperation.vi" "Left Ball Color"(w365) -> ()
    n227 = And(x=w352, y=w353) -> (x .and. y?=→"Has 2 Balls":bool)
    n228 = Wait (ms)(milliseconds to wait=u32 100) -> ()  [unwired: 1 out]
  }
  n229 = while {
    stop <- FALSE stop-if-true
    # "Intakes"
    # "Anti Jam"
    n230 = global read "ActuatorsSensors.vi" "Intake - F Output"() -> (w491:dbl)
    n231 = call <vilib>:"WPI_Power Get PDP Currents.vi"("PDP Channel"=8) -> ("current (A)"=w486:dbl)  [unwired: 12 in, 2 out]
    n232 = call <vilib>:"WPI_Power Get PDP Currents.vi"("PDP Channel"=7) -> ("current (A)"=w495:dbl)  [unwired: 12 in, 2 out]
    n233 = global read "ActuatorsSensors.vi" "Intake - R Output"() -> (w482:dbl)
    n234 = Greater?(x=w486, y=32.0) -> (0:w484:bool)
    n235 = Greater?(x=w495, y=30.0) -> (0:w494:bool)
    n236 = Select(t=1.0 ("f"), s=w484, f=w482) -> (s? t:f=w481:dbl)
    n237 = Select(t=-1.0 ("f"), s=w494, f=w491) -> (s? t:f=w490:dbl)
    n238 = global write "ActuatorsSensors.vi" "Intake - R Output No Jam"(w481) -> ()
    n239 = global write "ActuatorsSensors.vi" "Intake - F Output No Jam"(w490) -> ()
    n240 = Wait (ms)(milliseconds to wait=u32 100) -> ()  [unwired: 1 out]
  }
  n241 = while {
    stop <- FALSE stop-if-true
    n242 = global read "StateMachineOperation.vi" "Right Ball Color"() -> (w515:string)
    n243 = global read "StateMachineOperation.vi" "Left Ball Color"() -> (w517:string)
    n244 = global read "StateMachineOperation.vi" "Ball Color"() -> (w519:string)
    n245 = call-poly <vilib>:"NT Write Value.vi"("String"=w519, "Name"="Alliance") -> ()  [unwired: 9 in, 1 out]
    n246 = call-poly <vilib>:"NT Write Value.vi"("String"=w517, "Name"="Left Ball Color") -> ()  [unwired: 9 in, 1 out]
    n247 = call-poly <vilib>:"NT Write Value.vi"("String"=w515, "Name"="Right Ball Color") -> ()  [unwired: 9 in, 1 out]
    n248 = local read "Setpoint Shooter"() -> (w509:dbl)
    n249 = local read "ShooterRPM"() -> (w513:dbl)
    n250 = local read "RightColor"() -> (w506:u32)
    n251 = global read "Axes_N_Buttons.vi" "DrButtonB"() -> (w521:bool)
    n252 = local read "LeftColor"() -> (w508:u32)
    n253 = call-poly <vilib>:"NT Write Value.vi"("Boolean"=w521, "Name"="B Button") -> ()  [unwired: 9 in, 1 out]
    n254 = call-poly <vilib>:"NT Write Value.vi"("Numeric"=w513, "Name"="Shooter RPM") -> ()  [unwired: 9 in, 1 out]
    n255 = call-poly <vilib>:"NT Write Value.vi"("Numeric"=w509, "Name"="ShooterSP") -> ()  [unwired: 9 in, 1 out]
    n256 = call-poly <vilib>:"NT Write Value.vi"("Numeric"=w508, "Name"="LeftColor") -> ()  [unwired: 9 in, 1 out]
    n257 = call-poly <vilib>:"NT Write Value.vi"("Numeric"=w506, "Name"="RightColor") -> ()  [unwired: 9 in, 1 out]
    n258 = local read "Right Infrared Conveyor"() -> (w503:bool)
    n259 = local read "Left Infrared Conveyor"() -> (w502:bool)
    n260 = local read "Right Switch Conveyor"() -> (w501:bool)
    n261 = local read "Left Switch Conveyor"() -> (w504:bool)
    n262 = call-poly <vilib>:"NT Write Value.vi"("Boolean"=w504, "Name"="LeftSwitch") -> ()  [unwired: 9 in, 1 out]
    n263 = call-poly <vilib>:"NT Write Value.vi"("Boolean"=w503, "Name"="LeftIR") -> ()  [unwired: 9 in, 1 out]
    n264 = call-poly <vilib>:"NT Write Value.vi"("Boolean"=w502, "Name"="RightIR") -> ()  [unwired: 9 in, 1 out]
    n265 = call-poly <vilib>:"NT Write Value.vi"("Boolean"=w501, "Name"="RightSwitch") -> ()  [unwired: 9 in, 1 out]
    n266 = Wait (ms)(milliseconds to wait=u32 100) -> ()  [unwired: 1 out]
  }
  n267 = while {
    stop <- FALSE stop-if-true
    # "LED Control"
    n268 = local read "Opposite Ball Right"() -> (w549:bool)
    n269 = local read "RPM Ready?"() -> (w546:bool)
    n270 = local read "Opposite Ball Left"() -> (w552:bool)
    n271 = local read "Shooting?"() -> (w547:bool)
    n272 = local read "Has Ball Right"() -> (w548:bool)
    n273 = local read "Has Ball Left"() -> (w551:bool)
    n274 = global read "Robot Global Data.vi" "Robot Mode"() -> (w525:T20)
    n275 = call <vilib>:"WPI_DriverStationGetRemainingMatchTime.vi"() -> ("Match Time(s)"=w532:sgl)  [unwired: 10 in, 1 out]
    n276 = case shown="False" w547 {
      tunnel: [FALSE ("DIO 4") w576] -> w544
      tunnel: [FALSE ("DIO 5") w575] -> w545
      tunnel: w546 -> [_ w574]
      frame False {
      }
      frame True {
        n277 = case shown="True" w574 {
          tunnel: [TRUE ("DIO 4") FALSE ("DIO 4")] -> w576
          tunnel: [FALSE ("DIO 5") TRUE ("DIO 5")] -> w575
          frame False {
          }
          frame True {
          }
        }
      }
    }
    n278 = And(x=w551, y=w552) -> (x .and. y?=w553:bool)
    n279 = And(x=w548, y=w549) -> (x .and. y?=w550:bool)
    n280 = Equal?(x=w525, y=WPI_DriverStationRobotMode2."Autonomous Disabled" ("Robot Mode")) -> (x = y?=w523:bool)
    n281 = case shown="False" w553 {
      tunnel: [w590 TRUE ("DIO 1")] -> w542
      tunnel: [w591 FALSE ("DIO 0")] -> w543
      tunnel: w551 -> [w592 _]
      frame False {
        n282 = case shown="False" w592 {
          tunnel: [TRUE ("DIO 0") TRUE ("DIO 0")] -> w591
          tunnel: [TRUE ("DIO 1") FALSE ("DIO 1")] -> w590
          frame False {
          }
          frame True {
          }
        }
      }
      frame True {
      }
    }
    n283 = case shown="False" w550 {
      tunnel: [w581 TRUE ("DIO 1")] -> w539
      tunnel: [w582 FALSE ("DIO 0")] -> w541
      tunnel: w548 -> [w583 _]
      frame False {
        n284 = case shown="False" w583 {
          tunnel: [TRUE ("DIO 0") TRUE ("DIO 0")] -> w582
          tunnel: [TRUE ("DIO 1") FALSE ("DIO 1")] -> w581
          frame False {
          }
          frame True {
          }
        }
      }
      frame True {
      }
    }
    n285 = Less Or Equal?(x=w532, y=sgl 20.0) -> (x <= y?=w530:bool)
    n286 = Greater?(x=w532, y=sgl 0.0) -> (0:w529:bool)
    n287 = And(x=w530, y=w529) -> (x .and. y?=w528:bool)
    n288 = case shown="True" w528 {
      tunnel: w545 -> [w569 _]
      tunnel: [w569 TRUE ("DIO 5")] -> w535
      tunnel: w544 -> [w568 _]
      tunnel: [w568 TRUE ("DIO 4")] -> w537
      frame False {
      }
      frame True {
      }
    }
    n289 = case shown="False" w523 {
      tunnel: w543 -> [w560 _]
      tunnel: w542 -> [w561 _]
      tunnel: [w561 FALSE ("DIO 1")] -> w526
      tunnel: [w560 FALSE ("DIO 0")] -> w527
      tunnel: [w559 FALSE ("DIO 0")] -> w540
      tunnel: w541 -> [w559 _]
      tunnel: [w558 FALSE ("DIO 1")] -> w538
      tunnel: w539 -> [w558 _]
      tunnel: [w557 FALSE ("DIO 4")] -> w536
      tunnel: w537 -> [w557 _]
      tunnel: w535 -> [w556 _]
      tunnel: [w556 FALSE ("DIO 5")] -> w534
      frame False {
      }
      frame True {
      }
    }
    n290 = global write "ActuatorsSensors.vi" "DIO 4"(w536) -> ()
    n291 = global write "ActuatorsSensors.vi" "DIO 5"(w534) -> ()
    n292 = global write "ActuatorsSensors.vi" "DIO 0"(w540) -> ()
    n293 = global write "ActuatorsSensors.vi" "DIO 1"(w538) -> ()
    n294 = global write "ActuatorsSensors.vi" "DIO 2"(w527) -> ()
    n295 = global write "ActuatorsSensors.vi" "DIO 3"(w526) -> ()
    n296 = Wait (ms)(milliseconds to wait=u32 50) -> ()  [unwired: 1 out]
  }
  n297 = while {
    shift-right: [w626] -> _
    shift-left: _ -> [w625]
    shift-right: [w610] -> _
    shift-left: 0.0 ("y") -> [w611]
    stop <- FALSE stop-if-true
    # "Ball Control Routine"
    n298 = local read "Opposite Ball Right"() -> (w601:bool)
    n299 = local read "Opposite Ball Left"() -> (w600:bool)
    n300 = disable-structure shown="Enabled" {
      disable-tunnel: [w633 FALSE ("Toggled")] -> w604
      frame Disabled {
        n301 = global read "Axes_N_Buttons.vi" "OpLeft"() -> (w634:bool)
        n302 = call "Toggle.vi"("Initial Value"=FALSE, "In"=w634) -> ("Toggled"=w633:bool)  [unwired: 9 in]
      }
      frame Enabled {
      }
    }
    n303 = global read "Axes_N_Buttons.vi" "OpButtonRB"() -> (w627:bool)
    n304 = global read "Axes_N_Buttons.vi" "OpButtonLB"() -> (w628:bool)
    n305 = global read "Axes_N_Buttons.vi" "OpButtonA"() -> (w631:bool)
    n306 = global read "Axes_N_Buttons.vi" "OpButtonB"() -> (w630:bool)
    n307 = global read "Axes_N_Buttons.vi" "OpButtonY"() -> (w629:bool)
    n308 = global read "Axes_N_Buttons.vi" "OpButtonX"() -> (w616:bool)
    n309 = local read "Climbing?"() -> (w621:bool)
    n310 = Or(x=w600, y=w601) -> (x .or. y?=w599:bool)
    n311 = case shown="\"Shoot\"" w625 {
      tunnel: [w667 _ _ _ w762 w772 _ w824 _ 1.0 ("f")] -> w618
      tunnel: [w667 -1.0 ("Intake Front Output") -1.0 ("Intake Front Output") _ _ _ _ _ _ _] -> w620
      tunnel: w631 -> [w666 _ w699 w716 _ _ _ _ w835 _]
      tunnel: w630 -> [w662 w677 _ w713 _ _ _ _ w834 _]
      tunnel: w629 -> [_ w673 w689 w706 w770 w783 _ _ _ w852]
      tunnel: w628 -> [w659 _ _ _ _ _ _ _ _ _]
      tunnel: w627 -> [_ _ _ _ w761 _ _ _ w831 _]
      tunnel: [w669 w680 w698 w717 w768 w784 w807 w826 w829 w853] -> w626
      tunnel: [w651 _ _ _ TRUE TRUE _ TRUE _ TRUE] -> w624
      tunnel: [w651 TRUE TRUE _ _ _ _ _ _ TRUE] -> w613
      tunnel: w621 -> [w665 _ _ _ _ _ w812 _ w836 _]
      tunnel: [w667 _ _ _ w763 1.0 ("Intake Front Output") _ w823 _ 1.0 ("f")] -> w617
      tunnel: [w667 1.0 ("Intake Front Output") _ 1.0 ("Intake Front Output") _ _ _ _ _ _] -> w619
      tunnel: w616 -> [w660 w678 w697 _ _ _ _ _ w833 _]
      tunnel: [_ TRUE ("Intake - R Solenoid") _ TRUE ("Intake - R Solenoid") _ _ _ _ _ TRUE ("Intake - R Solenoid")] -> w615
      tunnel: w599 -> [w652 _ _ _ _ _ _ _ w830 _]
      tunnel: [w643 _ _ _ w729 w780 _ 600.0 ("Setpoint Shooter") _ 600.0 ("Setpoint Shooter")] -> w614
      tunnel: [w651 _ _ _ TRUE ("Compressor Off") TRUE ("Compressor Off") _ _ _ _] -> w612
      tunnel: w611 -> [_ _ _ _ _ w777 _ w816 _ _]
      tunnel: [0.0 _ _ _ 0.0 w778 _ w817 _ _] -> w610
      tunnel: [_ _ _ _ TRUE ("Overwrite Solenoid") _ _ _ _ _] -> w609
      tunnel: [w650 _ _ _ _ _ _ w818 _ _] -> w608
      tunnel: [w649 _ _ _ _ _ _ w819 _ _] -> w607
      tunnel: [_ _ _ _ w721 TRUE _ _ _ _] -> w606
      tunnel: [_ _ _ _ TRUE ("Shooting?") TRUE ("Shooting?") _ _ _ TRUE ("Shooting?")] -> w605
      tunnel: w604 -> [w647 w676 w690 w705 _ _ _ _ w832 _]
      tunnel: [w644 _ _ _ w730 w774 _ 1000.0 ("Setpoint Shooter Hood") _ _] -> w603
      tunnel: [w637 _ _ _ w728 _ _ _ _ _] -> w602
      frame "Default", Default {
        w651 = FALSE
        w667 = 0.0 ("Intake Front Output")
        n312 = Select(t=Ball_Routine_States."Default" ("Enum"), s=w647, f=Ball_Routine_States."Default" ("Enum")) -> (s? t:f=w645:T25)
        n313 = Select(t=Ball_Routine_States."Default" ("Enum"), s=w652, f=w645) -> (s? t:f=w654:T25)
        n314 = local read "Has Ball Right"() -> (w639:bool)
        n315 = local read "Has Ball Left"() -> (w640:bool)
        n316 = local read "Has 2 Balls"() -> (w642:bool)
        n317 = Select(t=Ball_Routine_States."Prepare Shooter" ("Enum"), s=w659, f=w654) -> (s? t:f=w658:T25)
        n318 = Or(x=w640, y=w639) -> (x .or. y?=w638:bool)
        n319 = Select(t=Ball_Routine_States."Rear Intake Collect" ("Enum"), s=w660, f=w658) -> (s? t:f=w657:T25)
        n320 = Select(t=FALSE, s=w642, f=w638) -> (s? t:f=w637:bool)
        n321 = Select(t=Ball_Routine_States."Front Intake Collect" ("Enum"), s=w662, f=w657) -> (s? t:f=w663:T25)
        n322 = local read "Hood Setpoint Shooter"() -> (w644:dbl)
        n323 = Select(t=Ball_Routine_States."Dual Intake Collect" ("Enum"), s=w666, f=w663) -> (s? t:f=w670:T25)
        n324 = local read "Opposite Ball Right"() -> (w649:bool)
        n325 = local read "Opposite Ball Left"() -> (w650:bool)
        n326 = Select(t=Ball_Routine_States."Climbing" ("Enum"), s=w665, f=w670) -> (s? t:f=w669:T25)
        n327 = local read "SpShooter"() -> (w643:dbl)
      }
      frame "Dual Intake Collect" {
        n328 = And(x=w673, y=w676) -> (x .and. y?=w675:bool)
        n329 = Select(t=Ball_Routine_States."Default" ("Enum"), s=w673, f=Ball_Routine_States."Dual Intake Collect" ("Enum")) -> (s? t:f=w671:T25)
        n330 = Select(t=Ball_Routine_States."Low Goal Mode" ("Enum"), s=w675, f=w671) -> (s? t:f=w684:T25)
        n331 = Select(t=Ball_Routine_States."Rear Intake Collect" ("Enum"), s=w678, f=w684) -> (s? t:f=w683:T25)
        n332 = Select(t=Ball_Routine_States."Front Intake Collect" ("Enum"), s=w677, f=w683) -> (s? t:f=w680:T25)
      }
      frame "Front Intake Collect" {
        n333 = And(x=w689, y=w690) -> (x .and. y?=w695:bool)
        n334 = Select(t=Ball_Routine_States."Default" ("Enum"), s=w689, f=Ball_Routine_States."Front Intake Collect" ("Enum")) -> (s? t:f=w691:T25)
        n335 = Select(t=Ball_Routine_States."Low Goal Mode" ("Enum"), s=w695, f=w691) -> (s? t:f=w692:T25)
        n336 = Select(t=Ball_Routine_States."Rear Intake Collect" ("Enum"), s=w697, f=w692) -> (s? t:f=w702:T25)
        n337 = Select(t=Ball_Routine_States."Dual Intake Collect" ("Enum"), s=w699, f=w702) -> (s? t:f=w698:T25)
      }
      frame "Rear Intake Collect" {
        n338 = And(x=w706, y=w705) -> (x .and. y?=w711:bool)
        n339 = Select(t=Ball_Routine_States."Default" ("Enum"), s=w706, f=Ball_Routine_States."Rear Intake Collect" ("Enum")) -> (s? t:f=w708:T25)
        n340 = Select(t=Ball_Routine_States."Low Goal Mode" ("Enum"), s=w711, f=w708) -> (s? t:f=w707:T25)
        n341 = Select(t=Ball_Routine_States."Front Intake Collect" ("Enum"), s=w713, f=w707) -> (s? t:f=w720:T25)
        n342 = Select(t=Ball_Routine_States."Dual Intake Collect" ("Enum"), s=w716, f=w720) -> (s? t:f=w717:T25)
      }
      frame "Prepare Shooter" {
        n343 = local read "Setpoint Shooter Hood"() -> (w725:dbl)
        n344 = local read "ShooterHoodRPM;"() -> (w724:dbl)
        n345 = local read "Setpoint Shooter"() -> (w758:dbl)
        n346 = global read "Axes_N_Buttons.vi" "OpAxis3"() -> (w747:dbl)
        n347 = local read "ShooterRPM"() -> (w760:dbl)
        n348 = Subtract(x=w758, y=20.0) -> (x-y=w757:dbl)
        n349 = Greater Or Equal?(x=w760, y=w757) -> (x >= y?=w727:bool)
        n350 = Greater?(x=w747, y=0.75) -> (0:w738:bool)
        n351 = Greater Or Equal?(x=w724, y=w725) -> (x >= y?=w726:bool)
        n352 = And(x=w727, y=w726) -> (x .and. y?=w721:bool)
        n353 = And(x=w761, y=w721) -> (x .and. y?=w722:bool)
        n354 = Select(t="SpShooter Low Goal", s=w738, f="SpShooter") -> (s? t:f=w733:dbl)
        n355 = Select(t=Ball_Routine_States."Default" ("Enum"), s=w770, f=Ball_Routine_States."Prepare Shooter" ("Enum")) -> (s? t:f=w769:T25)
        n356 = local read "Right Switch Conveyor"() -> (w742:bool)
        n357 = global read "ActuatorsSensors.vi" "IRS Right"() -> (w744:bool)
        n358 = global read "ActuatorsSensors.vi" "IRS Left"() -> (w743:bool)
        n359 = local read "Left Switch Conveyor"() -> (w745:bool)
        n360 = local read "1 Ball only"() -> (w736:bool)
        n361 = Select(t=Ball_Routine_States."Shoot" ("Enum"), s=w722, f=w769) -> (s? t:f=w768:T25)
        n362 = Or(x=w744, y=w745) -> (x .or. y?=w751:bool)
        n363 = Select(t="Hood Low Goal SP", s=w738, f="Hood Setpoint Shooter") -> (s? t:f=w731:dbl)
        n364 = Or(x=w742, y=w743) -> (x .or. y?=w748:bool)
        n365 = Select(t=0.0, s=w736, f=0.0) -> (s? t:f=w732:dbl)
        n366 = Select(t=0.0, s=w751, f=0.7) -> (s? t:f=w763:dbl)
        n367 = Select(t=0.0, s=w748, f=0.7) -> (s? t:f=w762:dbl)
        n368 = local read "1 Ball only"() -> (w728:bool)
        n369 = Subtract(x=w731, y=w732) -> (x-y=w730:dbl)
        n370 = Subtract(x=w733, y=w732) -> (x-y=w729:dbl)
      }
      frame "Shoot" {
        n371 = disable-structure shown="Enabled" {
          disable-tunnel: w777 -> [w786 w796]
          disable-tunnel: [w785 w794] -> w772
          frame Disabled {
            n372 = disable-structure shown="Enabled" {
              disable-tunnel: w786 -> [w792 _]
              disable-tunnel: [w791 0.8 ("f")] -> w785
              frame Enabled {
                n373 = Greater?(x=w792, y=4.0) -> (0:w787:bool)
                n374 = Select(t=1.0 ("Intake Front Output"), s=w787, f=0.0) -> (s? t:f=w791:dbl)
              }
              frame Disabled {
              }
            }
          }
          frame Enabled {
            n375 = Greater?(x=w796, y=4.0) -> (0:w795:bool)
            n376 = case shown="True" w795 {
              tunnel: [0.0 ("t") w802] -> w794
              frame False {
              }
              frame True {
                n377 = local read "Setpoint Shooter Hood"() -> (w806:dbl)
                n378 = local read "ShooterHoodRPM;"() -> (w800:dbl)
                n379 = Subtract(x=w806, y=0.0) -> (x-y=w799:dbl)
                n380 = Greater Or Equal?(x=w800, y=w799) -> (x >= y?=w803:bool)
                n381 = Select(t=1.0, s=w803, f=0.0) -> (s? t:f=w802:dbl)
              }
            }
          }
        }
        n382 = Select(t=Ball_Routine_States."Default" ("Enum"), s=w783, f=Ball_Routine_States."Shoot" ("Enum")) -> (s? t:f=w784:T25)
        n383 = Increment(x=w777) -> (x+1=w778:dbl)
        n384 = local read "Setpoint Shooter"() -> (w780:dbl)
        n385 = local read "Setpoint Shooter Hood"() -> (w774:dbl)
      }
      frame "Climbing" {
        n386 = Equal?(x=w812, y=FALSE) -> (x = y?=w810:bool)
        n387 = Select(t=Ball_Routine_States."Default" ("Enum"), s=w810, f=Ball_Routine_States."Climbing" ("Enum")) -> (s? t:f=w807:T25)
      }
      frame "Opposite Ball Detected" {
        w822 = 0.0 ("f")
        w825 = 1.0 ("Intake Front Output")
        n388 = Greater?(x=w816, y=15.0) -> (0:w814:bool)
        n389 = local read "Discard Right"() -> (w819:bool)
        n390 = local read "Discard Left"() -> (w818:bool)
        n391 = Select(t=Ball_Routine_States."Default" ("Enum"), s=w814, f=Ball_Routine_States."Opposite Ball Detected" ("Enum")) -> (s? t:f=w826:T25)
        n392 = Select(t=w825, s=w819, f=w822) -> (s? t:f=w823:dbl)
        n393 = Select(t=w825, s=w818, f=w822) -> (s? t:f=w824:dbl)
        n394 = Increment(x=w816) -> (x+1=w817:dbl)
      }
      frame "Low Goal Mode" {
        n395 = Select(t=Ball_Routine_States."Low Goal Mode" ("Enum"), s=w832, f=Ball_Routine_States."Default" ("Enum")) -> (s? t:f=w837:T25)
        n396 = Select(t=Ball_Routine_States."Opposite Ball Detected" ("Enum"), s=w830, f=w837) -> (s? t:f=w841:T25)
        n397 = Select(t=Ball_Routine_States."Low Goal Shoot" ("Enum"), s=w831, f=w841) -> (s? t:f=w845:T25)
        n398 = Select(t=Ball_Routine_States."Rear Intake Collect" ("Enum"), s=w833, f=w845) -> (s? t:f=w844:T25)
        n399 = Select(t=Ball_Routine_States."Front Intake Collect" ("Enum"), s=w834, f=w844) -> (s? t:f=w847:T25)
        n400 = Select(t=Ball_Routine_States."Dual Intake Collect" ("Enum"), s=w835, f=w847) -> (s? t:f=w850:T25)
        n401 = Select(t=Ball_Routine_States."Climbing" ("Enum"), s=w836, f=w850) -> (s? t:f=w829:T25)
      }
      frame "Low Goal Shoot" {
        n402 = Select(t=Ball_Routine_States."Low Goal Mode" ("Enum"), s=w852, f=Ball_Routine_States."Low Goal Shoot" ("Enum")) -> (s? t:f=w853:T25)
      }
    }
    "Setpoint Shooter" <- w614
    "Overwrite Solenoid" <- w609
    "Discard Right" <- w607
    "Discard Left" <- w608
    "Shooting?" <- w605
    "RPM Ready?" <- w606
    "Setpoint Shooter Hood" <- w603
    "1 Ball only" <- w602
    n403 = global write "ActuatorsSensors.vi" "Intake - F Output"(w620) -> ()
    n404 = global write "ActuatorsSensors.vi" "Intake - R Output"(w619) -> ()
    n405 = global write "ActuatorsSensors.vi" "Conveyor - L Output"(w618) -> ()
    n406 = global write "ActuatorsSensors.vi" "Conveyor - R Output"(w617) -> ()
    n407 = global write "StateMachineOperation.vi" "Enable Shooter"(w624) -> ()
    n408 = global write "ActuatorsSensors.vi" "Intake - F Solenoid"(w613) -> ()
    n409 = global write "ActuatorsSensors.vi" "Intake - R Solenoid"(w615) -> ()
    n410 = global write "ActuatorsSensors.vi" "Compressor Off"(w612) -> ()
    n411 = Wait (ms)(milliseconds to wait=u32 100) -> ()  [unwired: 1 out]
  }
  n412 = call <vilib>:"WPI_EncoderRefNum Registry Get.vi"("refnum name"="EncoderShooter") -> ("EncoderDevRef"=w1:T26)  [unwired: 9 in, 1 out]
  n413 = call <vilib>:"WPI_MotorControlRefNum Registry Get.vi"("refnum name"="Shooter") -> ("MotorControlDevRef"=w59:T6)  [unwired: 9 in, 1 out]
  n414 = call <vilib>:"CTRE_Phoenix_MotorControl_RefNumRegistryGet.vi"("refnum name"="HoodShooter") -> ("PhoenixMotorControlDevRef"=w3:T6)  [unwired: 9 in, 1 out]
  n415 = while {
    tunnel: w3 -> [w872]
    stop <- FALSE stop-if-true
    w885 = T29 0 items=["QuadEncoder"=0, "Analog"=2, "Tachometer"=4, "Pulse Width Encoded Position"=8, "Sensor Sum (S0 + S1)"=9, "Sensor Difference (D0 - D1)"=10, "Remote Source 0"=11, "Remote Source 1"=12, "Software Emulated"=15] ("Feedback Device")
    # "Hood Shooter PID Loop"
    n416 = local read "Setpoint Shooter Hood"() -> (w866:dbl)
    n417 = global read "StateMachineOperation.vi" "Enable Shooter"() -> (w867:bool)
    n418 = call <vilib>:"CTRE_Phoenix_MotorControl_ConfigClosedLoopRamp.vi"("secondsFromNeutralToFull"="Neutral to Full Seconds Hood", "PhoenixMotorControlDevRef"=w872) -> ("error out"=w887:errorcluster, "PhoenixMotorControlDevRef"=w888:T6)  [unwired: 8 in]
    n419 = call <vilib>:"CTRE_Phoenix_MotorControl_ConfigSelectedFeedbackSensor_Enhanced.vi"("error in (no error)"=w887, "Feedback Device"=w885, "PhoenixMotorControlDevRef"=w888) -> ("PhoenixMotorControlDevRef"=w884:T6)  [unwired: 7 in, 1 out]
    n420 = Not(x=w867) -> (.not. x?=w869:bool)
    n421 = Equal?(x=w866, y=0.0) -> (x = y?=w870:bool)
    n422 = call <vilib>:"CTRE_Phoenix_MotorControl_ConfigClosedLoopConstants.vi"("PhoenixMotorControlDevRef"=w884, "slotIdx"=0, "P"="P Hood", "I"="I Hood", "D"="D Hood", "F"="kF Hood", "I Zone"="I Zone Hood") -> ("PhoenixMotorControlDevRef"=w877:T6)  [unwired: 7 in, 1 out]
    n423 = Or(x=w870, y=w869) -> (x .or. y?=w868:bool)
    n424 = case shown="False" w868 {
      tunnel: w877 -> [w893 w902]
      tunnel: w866 -> [w891 _]
      frame False {
        w894 = T19 2 items=["PercentOutput"=0, "Position"=1, "Velocity"=2, "Current"=3, "Follower"=5, "MotionProfile"=6, "MotionMagic"=7, "MotionProfileArc"=10, "Disabled"=15] ("Control Mode")
        # "Converts RPM to Sensor Units"
        n425 = disable-structure shown="Enabled" {
          disable-tunnel: [w897 -1.0 ("Output")] -> w892
          disable-tunnel: w891 -> [w895 _]
          frame Enabled {
            n426 = Negate(x=w895) -> (-x=w896:dbl)
            n427 = Divide(x=w896, y=600.0 ("x")) -> (x/y=w899:dbl)
            n428 = Multiply(x=w899, y=8196.0) -> (x*y=w897:dbl)
          }
          frame Disabled {
          }
        }
        n429 = call <vilib>:"CTRE_Phoenix_MotorControl_Set.vi"("Output"=w892, "Control Mode"=w894, "PhoenixMotorControlDevRef"=w893) -> ()  [unwired: 7 in, 2 out]
      }
      frame True {
        w904 = T19 0 items=["PercentOutput"=0, "Position"=1, "Velocity"=2, "Current"=3, "Follower"=5, "MotionProfile"=6, "MotionMagic"=7, "MotionProfileArc"=10, "Disabled"=15] ("Control Mode")
        n430 = call <vilib>:"CTRE_Phoenix_MotorControl_Set.vi"("Output"=0.0, "Control Mode"=w904, "PhoenixMotorControlDevRef"=w902) -> ()  [unwired: 7 in, 2 out]
      }
    }
    n431 = call-poly <vilib>:"CTRE_Phoenix_MotorController_Get_Enhanced.vi"("PhoenixMotorControlDevRef"=w877) -> ("Velocity (Raw Sensor Units per 100 ms)"=w863:i32)  [unwired: 11 in, 3 out]
    n432 = Negate(x=w863) -> (-x=w862:i32)
    n433 = Divide(x=w862, y=8196.0) -> (x/y=w874:dbl)
    n434 = Multiply(x=600.0, y=w874) -> (x*y=w876:dbl)
    n435 = Negate(x=w876) -> (-x=w864:dbl)
    "ShooterHoodRPM;" <- w864
    n436 = Bundle("Setpoint Shooter Hood"=w866, w864) -> (→"Waveform Chart Hood":cluster{"Setpoint Shooter Hood":dbl, dbl})  [unwired: 1 in]
    n437 = Wait (ms)(milliseconds to wait=u32 20) -> ()  [unwired: 1 out]
  }
  n438 = while {
    tunnel: w59 -> [w915]
    shift-right: [w913] -> _
    shift-left: 0.0 ("y") -> [w914]
    tunnel: w1 -> [w905]
    stop <- FALSE stop-if-true
    # "Shooter PID"
    n439 = disable-structure shown="Enabled" {
      disable-tunnel: w915 -> [w930 w994]
      disable-tunnel: w914 -> [w922 _]
      disable-tunnel: [w921 _] -> w913
      disable-tunnel: [w920 w988] -> w912
      disable-tunnel: [w919 w979] -> w911
      disable-tunnel: [w918 w992] -> w910
      disable-tunnel: [w917 w993] -> w909
      disable-tunnel: [w916 w999] -> w908
      disable-tunnel: w905 -> [_ w983]
      frame Disabled {
        n440 = feedback #1() -> (w927:T3)  [unwired: 1 in]
        n441 = Not Equal?(x="PID Constants", y=w927) -> (x != y?=w924:T31)
        n442 = Cluster To Array(cluster=w924) -> (array=w923:bool[])
        n443 = Or Array Elements(Boolean array=w923) -> (logical OR=w925:bool)
        n444 = local read "Setpoint Shooter"() -> (w938:dbl)
        n445 = case shown="True" w925 {
          tunnel: w930 -> [w940 w943]
          tunnel: [w940 w942] -> w929
          tunnel: "PID Constants" -> [w939 w941]
          tunnel: [w939 w941] -> w928
          frame False {
          }
          frame True {
            n446 = call <vilib>:"Spark MAX Set PIDF Constants.vi"("PID Constants"=w941, "MotorControlDeviceRef"=w943) -> ("MotorControlDeviceRef"=w942:T6)  [unwired: 8 in, 1 out]
          }
        }
        n447 = feedback-in #1(w928) -> ()
        n448 = local read "Has 2 Balls"() -> (w933:bool)
        n449 = global read "StateMachineOperation.vi" "Enable Shooter"() -> (w937:bool)
        n450 = Select(t=Shooter_States."Cruise Velocity" ("Shooter States"), s=w933, f=Shooter_States."Disabled" ("Shooter States")) -> (s? t:f=w934:T30)
        n451 = Select(t=Shooter_States."Shooting Velocity" ("Shooter States"), s=w937, f=w934) -> (s? t:f=w935:T30)
        n452 = call <vilib>:"Spark MAX Get Sensor Velocity.vi"("MotorControlDevRef in"=w929) -> ("Sensor Velocity"=w919:dbl)  [unwired: 7 in, 3 out]
        n453 = call <vilib>:"Spark MAX Get Supply Current.vi"("MotorControlDevRef in"=w929) -> ()  [unwired: 7 in, 4 out]
        n454 = call <vilib>:"Spark MAX Get Supply Voltage.vi"("MotorControlDevRef in"=w929) -> ("Voltage"=w918:dbl)  [unwired: 7 in, 3 out]
        n455 = call <vilib>:"Spark MAX Get Applied Output.vi"("MotorControlDevRef in"=w929) -> ("Applied Output"=w920:dbl)  [unwired: 7 in, 3 out]
        n456 = case shown="\"Shooting Velocity\"" w935 {
          tunnel: w929 -> [w945 w951 w958]
          tunnel: w938 -> [_ _ w957]
          tunnel: w919 -> [_ _ w956]
          tunnel: w922 -> [_ _ w953]
          tunnel: [0.0 0.0 w954] -> w921
          frame "Disabled", Default {
            n457 = call <vilib>:"Spark MAX Set Output Advanced.vi"("Control Mode"=Spark_MAX_Control_Type."Percent VBus", "Setpoint"=0.0, "MotorControlDevRef"=w945) -> ()  [unwired: 7 in, 2 out]
          }
          frame "Cruise Velocity" {
            n458 = call <vilib>:"Spark MAX Set Output Advanced.vi"("Control Mode"=Spark_MAX_Control_Type."Velocity", "Setpoint"=600.0, "MotorControlDevRef"=w951) -> ()  [unwired: 7 in, 2 out]
          }
          frame "Shooting Velocity" {
            n459 = disable-structure shown="Enabled" {
              disable-tunnel: w957 -> [w970 _]
              disable-tunnel: w956 -> [w969 _]
              disable-tunnel: [w968 TRUE] -> w955
              disable-tunnel: [w967 _] -> w954
              disable-tunnel: w953 -> [w966 _]
              disable-tunnel: [w965 _] -> w952
              frame Enabled {
                n460 = Greater?(x=w966, y=1.0) -> (0:w959:bool)
                n461 = Select(t=1.0 ("y"), s=w959, f=0.9) -> (s? t:f=w965:dbl)
                n462 = Multiply(x=w970, y=0.8) -> (x*y=w963:dbl)
                n463 = Greater Or Equal?(x=w969, y=w963) -> (x >= y?=w968:bool)
                n464 = Increment(x=w966) -> (x+1=w967:dbl)
              }
              frame Disabled {
              }
            }
            n465 = case shown="True" w955 {
              tunnel: w958 -> [w974 w977]
              tunnel: w957 -> [_ w975]
              tunnel: w952 -> [w972 _]
              frame False {
                n466 = call <vilib>:"Spark MAX Set Output Advanced.vi"("Control Mode"=Spark_MAX_Control_Type."Percent VBus", "Setpoint"=w972, "MotorControlDevRef"=w974) -> ()  [unwired: 7 in, 2 out]
              }
              frame True {
                n467 = call <vilib>:"Spark MAX Set Output Advanced.vi"("Control Mode"=Spark_MAX_Control_Type."Velocity", "Setpoint"=w975, "MotorControlDevRef"=w977) -> ()  [unwired: 7 in, 2 out]
              }
            }
          }
        }
        n468 = Bundle("Applied Output"=w920) -> (w917:cluster{"Applied Output":dbl})  [unwired: 1 in]
        n469 = Bundle("Setpoint Shooter"=w938, "Sensor Velocity"=w919) -> (w916:T32)  [unwired: 1 in]
      }
      frame Enabled {
        n470 = local read "Has 2 Balls"() -> (w991:bool)
        n471 = global read "StateMachineOperation.vi" "Enable Shooter"() -> (w1003:bool)
        n472 = call <vilib>:"WPI_EncoderGet.vi"("EncoderDevRef"=w983) -> ("Rate"=w982:dbl)  [unwired: 5 in, 5 out]
        n473 = Select(t=Shooter_States."Cruise Velocity" ("Shooter States"), s=w991, f=Shooter_States."Disabled" ("Shooter States")) -> (s? t:f=w990:T30)
        n474 = Multiply(x=w982, y=60.0) -> (x*y=w980:dbl)
        n475 = Select(t=Shooter_States."Shooting Velocity" ("Shooter States"), s=w1003, f=w990) -> (s? t:f=w998:T30)
        n476 = case shown="\"Shooting Velocity\"" w998 {
          tunnel: [0.0 ("Setpoint") 600.0 ("Setpoint") w1009] -> w996
          tunnel: [FALSE ("s") TRUE ("s") TRUE ("s")] -> w985
          frame "Disabled", Default {
          }
          frame "Cruise Velocity" {
          }
          frame "Shooting Velocity" {
            n477 = local read "Setpoint Shooter"() -> (w1009:dbl)
          }
        }
        n478 = Negate(x=w980) -> (-x=w979:dbl)
        n479 = call "FancyPID.vi"("Gains"="Gains", "Range"="Range", "Integral Range"=10000.0, "Process variable"=w979, "Setpoint"=w996) -> ("output"=w987:dbl)  [unwired: 6 in]
        n480 = call <vilib>:"Spark MAX Get Supply Current.vi"("MotorControlDevRef in"=w994) -> ()  [unwired: 7 in, 4 out]
        n481 = call <vilib>:"Spark MAX Get Supply Voltage.vi"("MotorControlDevRef in"=w994) -> ("Voltage"=w992:dbl)  [unwired: 7 in, 3 out]
        n482 = call <vilib>:"Spark MAX Get Applied Output.vi"("MotorControlDevRef in"=w994) -> ("Applied Output"=w988:dbl)  [unwired: 7 in, 3 out]
        n483 = Select(t=w987, s=w985, f=0.0) -> (s? t:f=w978:dbl)
        n484 = Bundle("Applied Output"=w988) -> (w993:cluster{"Applied Output":dbl})  [unwired: 1 in]
        n485 = Bundle("Setpoint Shooter"=w996, w979) -> (w999:cluster{"Setpoint Shooter":dbl, dbl})  [unwired: 1 in]
        n486 = call <vilib>:"Spark MAX Set Output Advanced.vi"("Control Mode"=Spark_MAX_Control_Type."Percent VBus", "Setpoint"=w978, "MotorControlDevRef"=w994) -> ()  [unwired: 7 in, 2 out]
      }
    }
    "PID" <- w908
    "Output" <- w909
    "Voltage" <- w910
    "ShooterRPM" <- w911
    "Applied Output" <- w912
    n487 = Wait (ms)(milliseconds to wait=u32 10) -> ()  [unwired: 1 out]
  }
